vi "Core.vi"(0 "Image In":T12(plugin-control), 1 "CalibratedImage In":T12(plugin-control), 2 "Measurement JSON Data":T9 {"Ref ROI Cluster"."Edge Options ROI Ref"."Edge Polarity" items=["All Edges", "Rising Edges", "Falling Edges"]; "Ref ROI Cluster"."Edge Options ROI Ref"."Minimum Edge Strength" format="%.2f"; "Ref ROI Cluster"."Edge Options ROI Ref"."Width" step=2; "Ref ROI Cluster"."Edge Options ROI Ref"."Kernel Size" step=2; "Ref ROI Cluster"."Line Options ROI Ref"."Min. Points (%)" min=0.0 max=100.0; "Ref ROI Cluster"."Line Options ROI Ref"."Min. SNR (db)" min=0.0; "Ref ROI Cluster"."Line Options ROI Ref"."Max. Score" min=0.0 max=1024.0; "Ref ROI Cluster"."Line Options ROI Ref"."Min. Score" min=0.0 max=1024.0 step=1.0; "Measurement ROI 1 Cluster"."Meas ROI 1"."Contours"."Type" items=["No Selection", "Point", "Line", "Rectangle", "Oval", "Polygon", "Freehand Region", "Annulus", "Unused2", "Unused3", "Broken Line", "Freehand Line", "Rotated Rectangle"]; "Measurement ROI 1 Cluster"."Edge Options ROI 1"."Edge Polarity" items=["All Edges", "Rising Edges", "Falling Edges"]; "Measurement ROI 1 Cluster"."Edge Options ROI 1"."Minimum Edge Strength" format="%.2f"; "Measurement ROI 1 Cluster"."Edge Options ROI 1"."Width" step=2; "Measurement ROI 1 Cluster"."Edge Options ROI 1"."Kernel Size" step=2; "Measurement ROI 1 Cluster"."Line Options ROI 1"."Min. Points (%)" min=0.0 max=100.0; "Measurement ROI 1 Cluster"."Line Options ROI 1"."Min. SNR (db)" min=0.0; "Measurement ROI 1 Cluster"."Line Options ROI 1"."Max. Score" min=0.0 max=1024.0; "Measurement ROI 1 Cluster"."Line Options ROI 1"."Min. Score" min=0.0 max=1024.0 step=1.0; "Measurement ROI 1 Cluster"."Circle Options ROI 1"."Edge Options"."Edge Polarity" items=["All Edges", "Rising Edges", "Falling Edges"]; "Measurement ROI 1 Cluster"."Circle Options ROI 1"."Edge Options"."Minimum Edge Strength" format="%.2f"; "Measurement ROI 1 Cluster"."Circle Options ROI 1"."Edge Options"."Width" step=2; "Measurement ROI 1 Cluster"."Circle Options ROI 1"."Edge Options"."Kernel Size" step=2; "Measurement ROI 2 Cluster"."Meas ROI 2"."Contours"."Type" items=["No Selection", "Point", "Line", "Rectangle", "Oval", "Polygon", "Freehand Region", "Annulus", "Unused2", "Unused3", "Broken Line", "Freehand Line", "Rotated Rectangle"]; "Measurement ROI 2 Cluster"."Edge Options ROI 2"."Edge Polarity" items=["All Edges", "Rising Edges", "Falling Edges"]; "Measurement ROI 2 Cluster"."Edge Options ROI 2"."Minimum Edge Strength" format="%.2f"; "Measurement ROI 2 Cluster"."Edge Options ROI 2"."Width" step=2; "Measurement ROI 2 Cluster"."Edge Options ROI 2"."Kernel Size" step=2; "Measurement ROI 2 Cluster"."Line Options ROI 2"."Min. Points (%)" min=0.0 max=100.0; "Measurement ROI 2 Cluster"."Line Options ROI 2"."Min. SNR (db)" min=0.0; "Measurement ROI 2 Cluster"."Line Options ROI 2"."Max. Score" min=0.0 max=1024.0; "Measurement ROI 2 Cluster"."Line Options ROI 2"."Min. Score" min=0.0 max=1024.0 step=1.0; "Measurement ROI 2 Cluster"."Circle Options ROI 2"."Edge Options"."Edge Polarity" items=["All Edges", "Rising Edges", "Falling Edges"]; "Measurement ROI 2 Cluster"."Circle Options ROI 2"."Edge Options"."Minimum Edge Strength" format="%.2f"; "Measurement ROI 2 Cluster"."Circle Options ROI 2"."Edge Options"."Width" step=2; "Measurement ROI 2 Cluster"."Circle Options ROI 2"."Edge Options"."Kernel Size" step=2}, 3 "Transformed ROI cluster":T3 {"ROI Ref [ After Transformation]"."Contours"."Type" items=["No Selection", "Point", "Line", "Rectangle", "Oval", "Polygon", "Freehand Region", "Annulus", "Unused2", "Unused3", "Broken Line", "Freehand Line", "Rotated Rectangle"]; "Measurement ROI 1 [After Transformation]"."Contours"."Type" items=["No Selection", "Point", "Line", "Rectangle", "Oval", "Polygon", "Freehand Region", "Annulus", "Unused2", "Unused3", "Broken Line", "Freehand Line", "Rotated Rectangle"]; "Measurement ROI 2 [After Transformation]"."Contours"."Type" items=["No Selection", "Point", "Line", "Rectangle", "Oval", "Polygon", "Freehand Region", "Annulus", "Unused2", "Unused3", "Broken Line", "Freehand Line", "Rotated Rectangle"]}, 4 "Coordinate Other Cluster":T4, 5 "error in (no error)":errorcluster, 6 "coordinate system":T1) -> (13 "Overlay Arrow Lines":T11, 14 "Numeric":sgl, 19 "error out":errorcluster)   [LabVIEW 2019, in "Algorithm.lvclass"]
uses:
  FrameworkOverrides/Algorithm.lvclass
  <vilib>/vision/Measure.llb/Edge Options.ctl
  <vilib>/vision/Measure.llb/Edge Polarity.ctl
  <vilib>/vision/Measure.llb/Straight Edge Options.ctl
  <vilib>/vision/Measure.llb/Straight Edge Process.ctl
  <vilib>/vision/NI_Vision_Development_Module.lvlib
panel:
  out "Circle Fit Options ROI 1":T10
  out "Real World Value":sgl
  out "Pixel Value":sgl
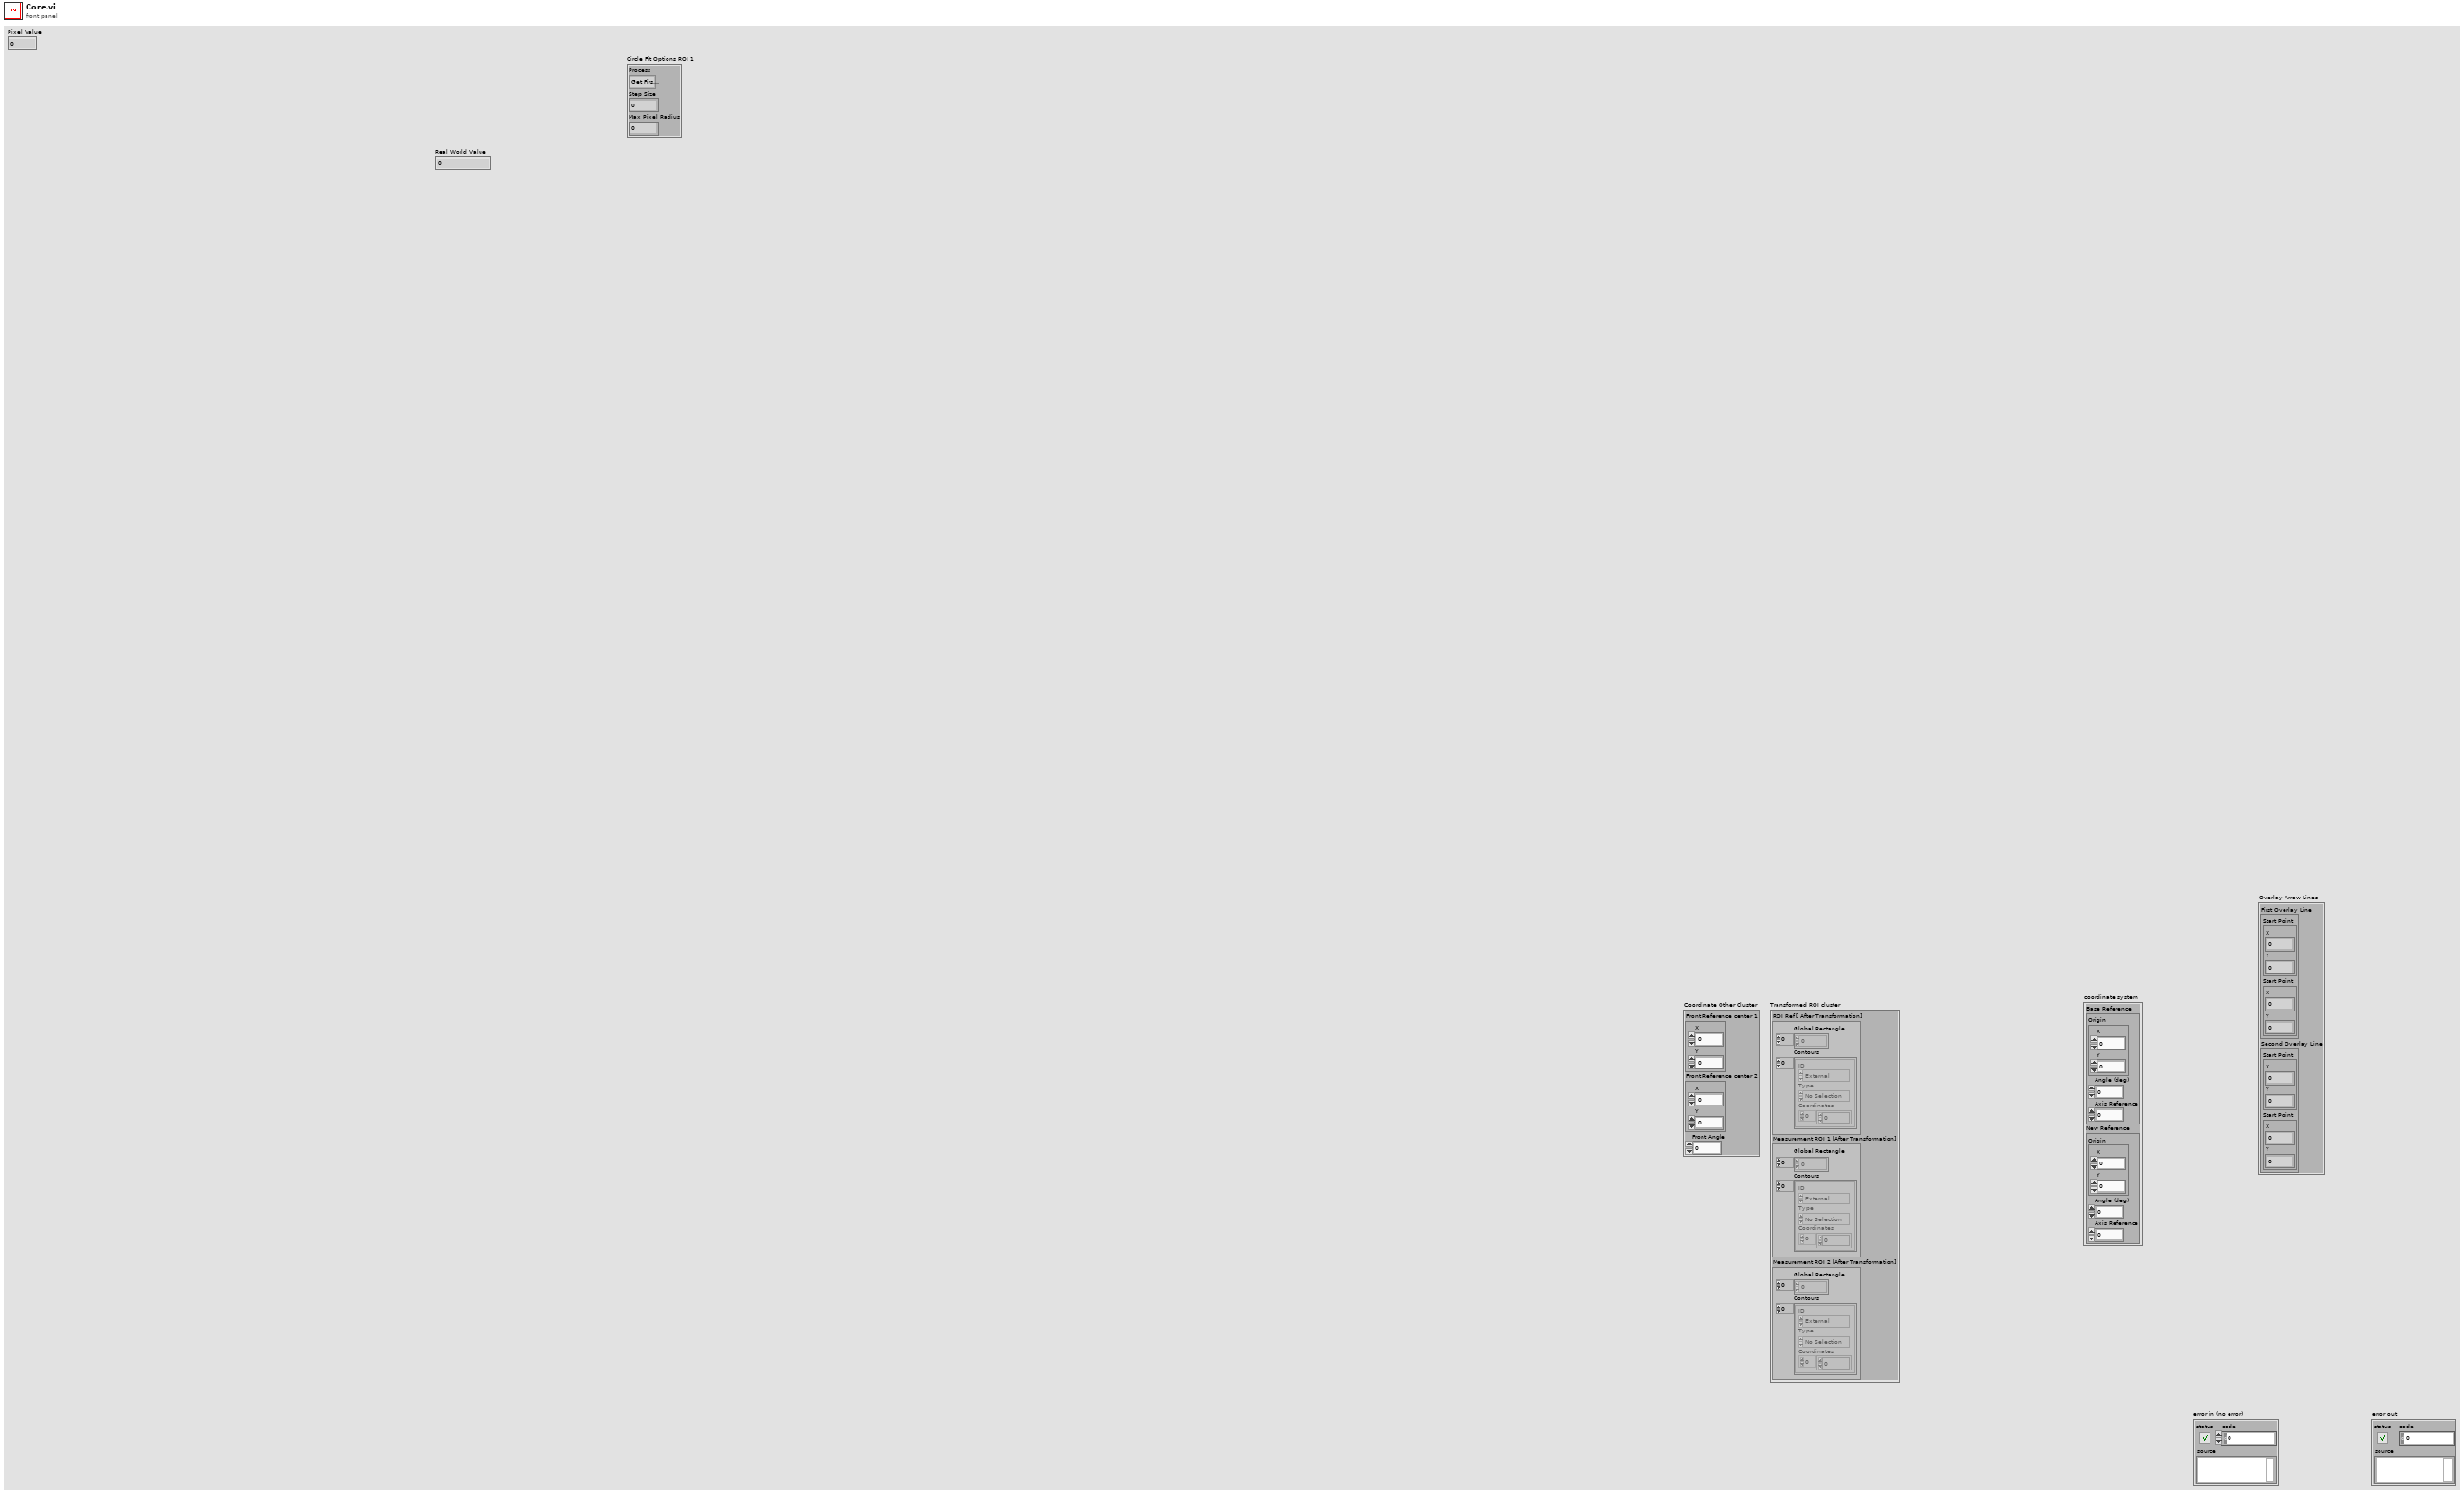
[diagram p1: front panel]
types:
  T1 = cluster{"Base Reference":cluster{"Origin":cluster{"X":sgl, "Y":sgl}, "Angle (deg)":sgl, "Axis Reference":u32}, "New Reference":cluster{"Origin":cluster{"X":sgl, "Y":sgl}, "Angle (deg)":sgl, "Axis Reference":u32}}
  T2 = typedef "ROI Descriptor" = cluster{"Global Rectangle":i32[], "Contours":cluster{"ID":enum32{"External", "Internal"}, "Type":u32, "Coordinates":i32[]}[]}
  T3 = cluster{"ROI Ref [ After Transformation]":T2, "Measurement ROI 1 [After Transformation]":T2, "Measurement ROI 2 [After Transformation]":T2}
  T4 = cluster{"Front Reference center 1":cluster{"X":sgl, "Y":sgl}, "Front Reference center 2":cluster{"X":sgl, "Y":sgl}, "Front Angle":dbl}
  T5 = typedef "Edge Options.ctl" = cluster{"Edge Polarity":T6, "Kernel Size":u32, "Width":u32, "Minimum Edge Strength":sgl, "Interpolation Type":enum32{"Zero Order", "Bilinear", "Quadratic", "Cubic", "Bilinear Fixed"}, "Data Processing Method":enum32{"Average", "Median"}}
  T6 = typedef "Edge Polarity.ctl" = u32
  T7 = typedef "Straight Edge Options.ctl" = cluster{"Number of Lines":i32, "Type":T8, "Min. Score":dbl, "Max. Score":dbl, "Orientation":dbl, "Angle Range":dbl, "Angle Tolerance":dbl, "Step Size":u32, "Min. SNR (db)":dbl, "Min. Points (%)":dbl, "Hough Iterations":i32}
  T8 = typedef "Straight Edge Process.ctl" = enum32{"First Edge Rake", "Best Edge Rake", "Hough Edge Rake", "First Edge Projection", "Best Edge Projection"}
  T9 = cluster{"RackID":i32, "ImageID":i32, "CameraID":i32, "MeasurementID":i32, "Measurement Name":string, "Algo Name":string, "Algo Type":string, "Ref ROI Cluster":cluster{"ROI Ref":cluster{"Global Rectangle":i32[], "Contours":cluster{"ID":enum32{"External", "Internal"}, "Type":u32, "Coordinates":i32[]}[]}, "Edge Options ROI Ref":T5, "Line Options ROI Ref":T7, "Search Direction ROI Ref":u32, "RefROIEnable":bool}, "Measurement ROI 1 Cluster":cluster{"Meas ROI 1":T2, "Edge Options ROI 1":T5, "Line Options ROI 1":T7, "Scan/Search Direction ROI 1":u16, "Step Size ROI 1":u32, "Process ROI 1":enum16{"Get First Edge", "Get First + Last Edge", "Get All Edges", "Get Best Edge"}, "Circle Options ROI 1":cluster{"Search  Direction":u32, "Edge Options":T5, "Show Search Area":bool, "Show Search Lines":bool, "Show Edges Found":bool, "Show Result":bool, "Search Area Color":u32, "Search Lines Color":u32, "Edge Locations Color":u32, "Result Color":u32, "Overlay Group Name":string}, "Circle Fit Options ROI 1":cluster{"Process":enum16{"Get First Edge", "Get First + Last Edge", "Get All Edges", "Get Best Edge"}, "Step Size":dbl, "Max Pixel Radius":i32}}, "Measurement ROI 2 Cluster":cluster{"Meas ROI 2":T2, "Edge Options ROI 2":T5, "Line Options ROI 2":T7, "Scan/Search Direction ROI 2":u32, "Step Size ROI 2":u32, "Process ROI 2":enum16{"Get First Edge", "Get First + Last Edge", "Get All Edges", "Get Best Edge"}, "Circle Options ROI 2":cluster{"Search  Direction":u32, "Edge Options":T5, "Show Search Area":bool, "Show Search Lines":bool, "Show Edges Found":bool, "Show Result":bool, "Search Area Color":u32, "Search Lines Color":u32, "Edge Locations Color":u32, "Result Color":u32, "Overlay Group Name":string}, "Circle Fit Options ROI 2":cluster{"Process":enum16{"Get First Edge", "Get First + Last Edge", "Get All Edges", "Get Best Edge"}, "Step Size":dbl, "Max Pixel Radius":i32}}, "OverlayOptions":cluster{"OverlayEnable":bool, "OverlayText":string, "OverlayCoords":i32[], "OverlayAngle":i32, "OverlayTextSize":i32, "OverlayTextColor":string, "OverlayROI":bool, "OverlayRakeLine":bool, "OverlayPoints":bool}, "MathExpression":cluster{"Algorithm":string, "MathExpression":string, "ResultVariable":string}, "MathCorrectionParameters":cluster{"Radius":dbl, "CurlGap":dbl, "Thickness":dbl, "MeasurementIndices":i32[], "MathAlgoName":string, "MathAlgoFormula":string, "CorrectionForAngle":i32[], "NumericAray":i32[], "StringArray":string[]}, "ResultVariableCluster":cluster{"RVName":string, "RVSequence":string, "RVIndex":i32, "RVID":i32, "RVValue":dbl}, "CalibrationCoefficients":cluster{"A1":dbl, "A2":dbl, "A3":dbl}, cluster{"UserCalibCoefficients":cluster{"UserCorrectionLinearityCoeff":dbl, "UserCorrectionBiasCoeff":dbl}}, "SpecValues":cluster{"LCL":dbl, "UCL":dbl, "LSL":dbl, "USL":dbl, "NominalValue":dbl}}
  T10 = cluster{"Process":enum16{"Get First Edge", "Get First + Last Edge", "Get All Edges", "Get Best Edge"}, "Step Size":dbl, "Max Pixel Radius":i32}
  T11 = cluster{"First Overlay Line ":cluster{"Start Point":cluster{"X":sgl, "Y":sgl}, "Start Point":cluster{"X":sgl, "Y":sgl}}, "Second Overlay Line ":cluster{"Start Point":cluster{"X":sgl, "Y":sgl}, "Start Point":cluster{"X":sgl, "Y":sgl}}}
  T12 = typedef "IMAQ Image.ctl" = refnum<image>
  T13 = cluster{"Contrast":i32, "Filter width":i32, "Steepness":i32, "Subsampling Ratio":u32, "Show Search Area":bool, "Show Search Lines":bool, "Show Edges Found":bool, "Show Result":bool}
  T14 = cluster{"AvgMinMax":enum16{"Average", "Max", "Min", "Max2"}, "Center X &Y":cluster{"Center X":dbl, "Center Y":dbl}, "Reference ROI Before Transformation":T2, "Measurement ROI-1 Before transformation":T2, "Ref Line Edge Options":T5, "Ref Line Search Direction":u32, "Ref Line Options":T7, "Meas ROI-1 Edge Options":T5, "Meas ROI-1 Step Size":u32, "Meas ROI-1 Scan Direction":u16, "Meas ROI-1 Process":enum16{"Get First Edge", "Get First + Last Edge", "Get All Edges", "Get Best Edge"}, "OverlayOptions":cluster{"OverlayEnable":bool, "OverlayText":string, "OverlayCoords":i32[], "OverlayAngle":i32, "OverlayTextSize":i32, "OverlayTextColor":string, "OverlayROI":bool, "OverlayRakeLine":bool, "OverlayPoints":bool}}
  T15 = cluster{"ROI 2 Descriptor":T2, " ROI 2 Step Size":u32, "ROI 2 Scan Direction":u16, "ROI 2 Process":enum16{"Get First Edge", "Get First + Last Edge", "Get All Edges", "Get Best Edge"}, "ROI 2 Edge Options":T5, "ROI 2 Overlay":bool, "ROI 2 Rake Line Overlay":bool, "ROI 2 Edge/Point Overlay":bool}
  T16 = cluster{"ROI 1 Descriptor":cluster{"Global Rectangle":i32[], "Contours":cluster{"ID":enum32{"External", "Internal"}, "Type":u32, "Coordinates":i32[]}[]}, "ROI 1 Line Options":T7, "ROI 1 Edge Options":T5, "ROI 1 Search Direction":u32, "ROI 1 Overlay":bool, "ROI 1 Rake Line Overlay":bool, "ROI 1 Edge/Point Overlay":bool}
  T17 = cluster{"ROI 2 After Transformation":cluster{"Global Rectangle":i32[], "Contours":cluster{"ID":enum32{"External", "Internal"}, "Type":u32, "Coordinates":i32[]}[]}, "ROI 2 Edge Options":T5, "ROI 2 Scan Direction":u16, "ROI 2 Step Size":u32, "ROI 2 Process":enum16{"Get First Edge", "Get First + Last Edge", "Get All Edges", "Get Best Edge"}, "ROI 2 Overlay":bool, "ROI 2 Rake Line Overlay":bool, "ROI 2 Edge/Point Overlay":bool}
  T18 = cluster{"ROI 1 After Transformation":cluster{"Global Rectangle":i32[], "Contours":cluster{"ID":enum32{"External", "Internal"}, "Type":u32, "Coordinates":i32[]}[]}, "ROI 1 Edge Options":T5, "ROI 1 Scan Direction":u16, "ROI 1 Step Size":u32, "ROI 1 Process":enum16{"Get First Edge", "Get First + Last Edge", "Get All Edges", "Get Best Edge"}, "ROI 1 Overlay":bool, "ROI 1 Rake Line Overlay":bool, "ROI 1 Edge/Point Overlay":bool}
  T19 = cluster{"Ref ROI After Transformation":cluster{"Global Rectangle":i32[], "Contours":cluster{"ID":enum32{"External", "Internal"}, "Type":u32, "Coordinates":i32[]}[]}, "Ref ROI Edge Options":T5, "Ref ROI Line Options":T7, "Ref ROI Search Direction":u32, "Ref ROI Overlay":bool}
  T20 = cluster{"Point 2":cluster{"X":sgl, "Y":sgl}, "Start Point":cluster{"X":sgl, "Y":sgl}}
  T21 = cluster{"Start Point":cluster{"X":sgl, "Y":sgl}, "Point 1":cluster{"X":sgl, "Y":sgl}}
  T22 = cluster{"First Overlay Line ":cluster{"Start Point":cluster{"X":sgl, "Y":sgl}, "Point 1":cluster{"X":sgl, "Y":sgl}}, "Second Overlay Line ":cluster{"Point 2":cluster{"X":sgl, "Y":sgl}, "Start Point":cluster{"X":sgl, "Y":sgl}}}
  T23 = cluster{"Search Direction":u32, "Edge Options":T5, "Show Search Area":bool, "Show Search Lines":bool, "Show Edges Found":bool, "Show Result":bool, "Search Area Color":u32, "Search Lines Color":u32, "Edge Locations Color":u32, "Result Color":u32, "Overlay Group Name":string}
  T24 = enum16{"Get First Edge", "Get First + Last Edge", "Get All Edges", "Get Best Edge"}
  T25 = cluster{"First Overlay Line ":cluster{"Start Point":cluster{"X":sgl, "Y":sgl}, "Intersection Point":cluster{"X":sgl, "Y":sgl}}, "Second Overlay Line ":cluster{"Intersection Point":cluster{"X":sgl, "Y":sgl}, "Start Point":cluster{"X":sgl, "Y":sgl}}}
  T26 = cluster{"First Overlay Line ":cluster{"Point 1":cluster{"X":sgl, "Y":sgl}, "Point 1":cluster{"X":sgl, "Y":sgl}}, "Second Overlay Line ":cluster{"Point 2":cluster{"X":sgl, "Y":sgl}, "Point 1":cluster{"X":sgl, "Y":sgl}}}
  T27 = cluster{"ROI 1 Before Transformation":cluster{"Global Rectangle":i32[], "Contours":cluster{"ID":enum32{"External", "Internal"}, "Type":u32, "Coordinates":i32[]}[]}, "ROI 1 Scan Direction":u16, "ROI 1 Edge Options":T5, "ROI 1Step Size":u32, "ROI 1 Process":enum16{"Get First Edge", "Get First + Last Edge", "Get All Edges", "Get Best Edge"}, "ROI 1 Overlay":bool, "ROI 1 Rake Line Overlay":bool, "ROI 1 Edge/Point Overlay":bool}
  T28 = cluster{"Ref Line ROI Before Transformation":cluster{"Global Rectangle":i32[], "Contours":cluster{"ID":enum32{"External", "Internal"}, "Type":u32, "Coordinates":i32[]}[]}, "Ref ROI Search Direction":u32, "Ref ROI Edge Options":T5, "Ref ROI Line Options":T7, "Ref ROI Overlay":bool, "Ref Rake Line Overlay 2":bool, "Ref Edge/Point Overlay":bool}
  T29 = cluster{"Overlay ROI":bool, "Overlay Edge/ Points":bool, "Overlay Rake Lines":bool}
  T30 = cluster{"1629 side E Ref ROI before transformation":T2, "Ref Search Direction":u32, "Ref Edge Options":T5, "Ref Line Options":T7, "Meas ROI-1 Descriptor before transformation":T2, "Meas-1 Step Size":u32, "Meas-1 Scan Direction":u16, "Meas-1 Edge Options":T5, "Meas ROI-2 Descriptor Before Transformation":T2, "Meas-2 Scan Direction":u32, "Meas-2 Edge Options":T5, "Meas-2 Line Options":T7, "Ellipse Center":cluster{"X":sgl, "Y":sgl}}
  T31 = cluster{"OverlayEnable":bool, "OverlayText":string, "OverlayCoords":i32[], "OverlayAngle":i32, "OverlayTextSize":i32, "OverlayTextColor":string, "OverlayROI":bool, "OverlayRakeLine":bool, "OverlayPoints":bool}
  T32 = typedef "Edge New.ctl" = cluster{"Location (Pixel)":cluster{"X":sgl, "Y":sgl}, "Location (Real-World)":cluster{"X":sgl, "Y":sgl}, "Distance (Pixel)":dbl, "Distance (Real-World)":dbl, "Strength":dbl, "Noise":dbl, "Rising?":bool}
  T33 = typedef "Search Line.ctl" = cluster{"Start Point":cluster{"X":sgl, "Y":sgl}, "End Point":cluster{"X":sgl, "Y":sgl}, "Edge Info":T32[], "Edge Map":dbl[], "Calibration Valid":bool}
  T34 = cluster{"Start Point":cluster{"X":sgl, "Y":sgl}, "Location (Pixel)":cluster{"X":sgl, "Y":sgl}, "Location (Pixel)":cluster{"X":sgl, "Y":sgl}, "End Point":cluster{"X":sgl, "Y":sgl}}
  T35 = typedef "IMAQ Rectangle" = cluster{"Left":i32, "Top":i32, "Right":i32, "Bottom":i32, "Rotation":dbl}
  T36 = cluster{"element":cluster{"X":sgl, "Y":sgl}, cluster{"X":sgl, "Y":sgl}, cluster{"X":sgl, "Y":sgl}, "element":cluster{"X":sgl, "Y":sgl}}
  T37 = cluster{"element":cluster{"X":sgl, "Y":sgl}, "element":cluster{"X":sgl, "Y":sgl}}
  T38 = cluster{"Origin":cluster{"X":sgl, "Y":sgl}, "Angle (deg)":sgl, "Axis Reference":u32}
  T39 = cluster{"Global Rectangle":i32[], "Contours":cluster{"ID":enum32{"External", "Internal"}, "Type":u32, "Coordinates":i32[]}[]}
  T40 = cluster{"L":dbl, "Line Coordinates":cluster{"Point1":cluster{"X":sgl, "Y":sgl}, "Point2":cluster{"X":sgl, "Y":sgl}}}
  T41 = cluster{"L Meas":sgl, "output cluster":cluster{"Point 2":cluster{"X":sgl, "Y":sgl}, "Point 2":cluster{"X":sgl, "Y":sgl}}}
  T42 = cluster{cluster{cluster{sgl, "Y":sgl}, "Point 2":cluster{"X":sgl, "Y":sgl}}, cluster{"Point 2":cluster{"X":sgl, "Y":sgl}, cluster{sgl, "Y":sgl}}}
  T43 = cluster{"Point1 (Pixels)":cluster{"X":sgl, "Y":sgl}, "Point2 (Pixels)":cluster{"X":sgl, "Y":sgl}, "Point1 (Real-World)":cluster{"X":sgl, "Y":sgl}, "Point2 (Real-World)":cluster{"X":sgl, "Y":sgl}, "Angle (Pixel)":dbl, "Angle (Real-World)":dbl, "Score":dbl, "Straightness":dbl, "Average SNR (db)":dbl, "Calibration Valid":bool}[]
  T44 = cluster{"Point1 (Pixels)":cluster{"X":sgl, "Y":sgl}, "Point2 (Pixels)":cluster{"X":sgl, "Y":sgl}, "Point1 (Real-World)":cluster{"X":sgl, "Y":sgl}, "Point2 (Real-World)":cluster{"X":sgl, "Y":sgl}, "Angle (Pixel)":dbl, "Angle (Real-World)":dbl, "Score":dbl, "Straightness":dbl, "Average SNR (db)":dbl, "Calibration Valid":bool}
  T45 = cluster{"Point1 (Pixels)":cluster{"X":sgl, "Y":sgl}, "Point2 (Pixels)":cluster{"X":sgl, "Y":sgl}}
  T46 = cluster{"Point 1":cluster{"X":sgl, "Y":sgl}, "Point 2":cluster{"X":sgl, "Y":sgl}}
  T47 = cluster{"Search  Direction":u32, "Edge Options":T5, "Show Search Area":bool, "Show Search Lines":bool, "Show Edges Found":bool, "Show Result":bool, "Search Area Color":u32, "Search Lines Color":u32, "Edge Locations Color":u32, "Result Color":u32, "Overlay Group Name":string}
  T48 = typedef "IMAQ Circle" = cluster{"Center X":i32, "Center Y":i32, "Inner Radius":i32, "Outer Radius":i32, "Start Angle":dbl, "End Angle":dbl}
  T49 = cluster{"Center (Pixels)":cluster{"X":sgl, "Y":sgl}, "Radius (Pixels)":dbl, "Center (Real-World)":cluster{"X":sgl, "Y":sgl}, "Radius (Real-World)":dbl, "Roundness (Real-World)":dbl, "Average Strength":dbl, "Average SNR (dB)":dbl}
  T50 = cluster{"Center (Pixels)":cluster{"X":sgl, "Y":sgl}, "Center (Pixels)":cluster{"X":sgl, "Y":sgl}}
  T51 = cluster{cluster{"Center (Pixels)":cluster{"X":sgl, "Y":sgl}, "Center (Pixels)":cluster{"X":sgl, "Y":sgl}}, cluster{"Center (Pixels)":cluster{"X":sgl, "Y":sgl}, "Center (Pixels)":cluster{"X":sgl, "Y":sgl}}}
  T52 = cluster{cluster{sgl, "Y":sgl}, cluster{"X":sgl, "Y":sgl}}
  T53 = cluster{cluster{"X":sgl, "Y":sgl}, cluster{sgl, "Y":sgl}}
  T54 = cluster{"Meas ROI 1":T2, "Edge Options ROI 1":T5, "Line Options ROI 1":T7, "Scan/Search Direction ROI 1":u16, "Step Size ROI 1":u32, "Process ROI 1":enum16{"Get First Edge", "Get First + Last Edge", "Get All Edges", "Get Best Edge"}, "Circle Options ROI 1":cluster{"Search  Direction":u32, "Edge Options":T5, "Show Search Area":bool, "Show Search Lines":bool, "Show Edges Found":bool, "Show Result":bool, "Search Area Color":u32, "Search Lines Color":u32, "Edge Locations Color":u32, "Result Color":u32, "Overlay Group Name":string}, "Circle Fit Options ROI 1":cluster{"Process":enum16{"Get First Edge", "Get First + Last Edge", "Get All Edges", "Get Best Edge"}, "Step Size":dbl, "Max Pixel Radius":i32}}
  T55 = cluster{"Meas ROI 2":T2, "Edge Options ROI 2":T5, "Line Options ROI 2":T7, "Scan/Search Direction ROI 2":u32, "Step Size ROI 2":u32, "Process ROI 2":enum16{"Get First Edge", "Get First + Last Edge", "Get All Edges", "Get Best Edge"}, "Circle Options ROI 2":cluster{"Search  Direction":u32, "Edge Options":T5, "Show Search Area":bool, "Show Search Lines":bool, "Show Edges Found":bool, "Show Result":bool, "Search Area Color":u32, "Search Lines Color":u32, "Edge Locations Color":u32, "Result Color":u32, "Overlay Group Name":string}, "Circle Fit Options ROI 2":cluster{"Process":enum16{"Get First Edge", "Get First + Last Edge", "Get All Edges", "Get Best Edge"}, "Step Size":dbl, "Max Pixel Radius":i32}}
  T56 = cluster{"ROI Ref":cluster{"Global Rectangle":i32[], "Contours":cluster{"ID":enum32{"External", "Internal"}, "Type":u32, "Coordinates":i32[]}[]}, "Edge Options ROI Ref":T5, "Line Options ROI Ref":T7, "Search Direction ROI Ref":u32, "RefROIEnable":bool}
  T57 = cluster{cluster{cluster{"X":sgl, sgl}, cluster{"X":sgl, "Y":sgl}}, cluster{"Location (Pixel)":cluster{"X":sgl, "Y":sgl}, cluster{"X":sgl, sgl}}}
  T58 = cluster{cluster{cluster{sgl, "Y":sgl}, "Intersection Point":cluster{"X":sgl, "Y":sgl}}, cluster{"Intersection Point":cluster{"X":sgl, "Y":sgl}, cluster{sgl, "Y":sgl}}}
  T59 = cluster{"E Side EMeasurement":sgl, "Points for Arrow Overlay":cluster{"X":sgl, "Y":sgl}[]}
  T60 = cluster{"End Point":cluster{"X":sgl, "Y":sgl}, "End Point":cluster{"X":sgl, "Y":sgl}}
  T61 = cluster{cluster{"End Point":cluster{"X":sgl, "Y":sgl}, "End Point":cluster{"X":sgl, "Y":sgl}}, cluster{"End Point":cluster{"X":sgl, "Y":sgl}, "End Point":cluster{"X":sgl, "Y":sgl}}}
  T62 = cluster{"Left":dbl, "Top":dbl, "Right":dbl, "Bottom":dbl, "Angle":dbl}
  T63 = cluster{cluster{"element":cluster{"X":sgl, "Y":sgl}, "element":cluster{"X":sgl, "Y":sgl}}, cluster{"element":cluster{"X":sgl, "Y":sgl}, "element":cluster{"X":sgl, "Y":sgl}}}
  T64 = cluster{cluster{cluster{"X":sgl, sgl}, "Point 1":cluster{"X":sgl, "Y":sgl}}, cluster{"Point 2":cluster{"X":sgl, "Y":sgl}, cluster{"X":sgl, sgl}}}
  T65 = cluster{"Points for Overlay":cluster{"X":sgl, "Y":sgl}[], "E1":sgl}
  T66 = cluster{"Point 1":cluster{"X":sgl, "Y":sgl}, "Point 1":cluster{"X":sgl, "Y":sgl}}
  T67 = cluster{cluster{"Point 1":cluster{"X":sgl, "Y":sgl}, "Point 1":cluster{"X":sgl, "Y":sgl}}, cluster{"Point 1":cluster{"X":sgl, "Y":sgl}, "Point 1":cluster{"X":sgl, "Y":sgl}}}
  T68 = cluster{cluster{cluster{sgl, "Y":sgl}, "Point 1":cluster{"X":sgl, "Y":sgl}}, cluster{"Point 2":cluster{"X":sgl, "Y":sgl}, cluster{sgl, "Y":sgl}}}
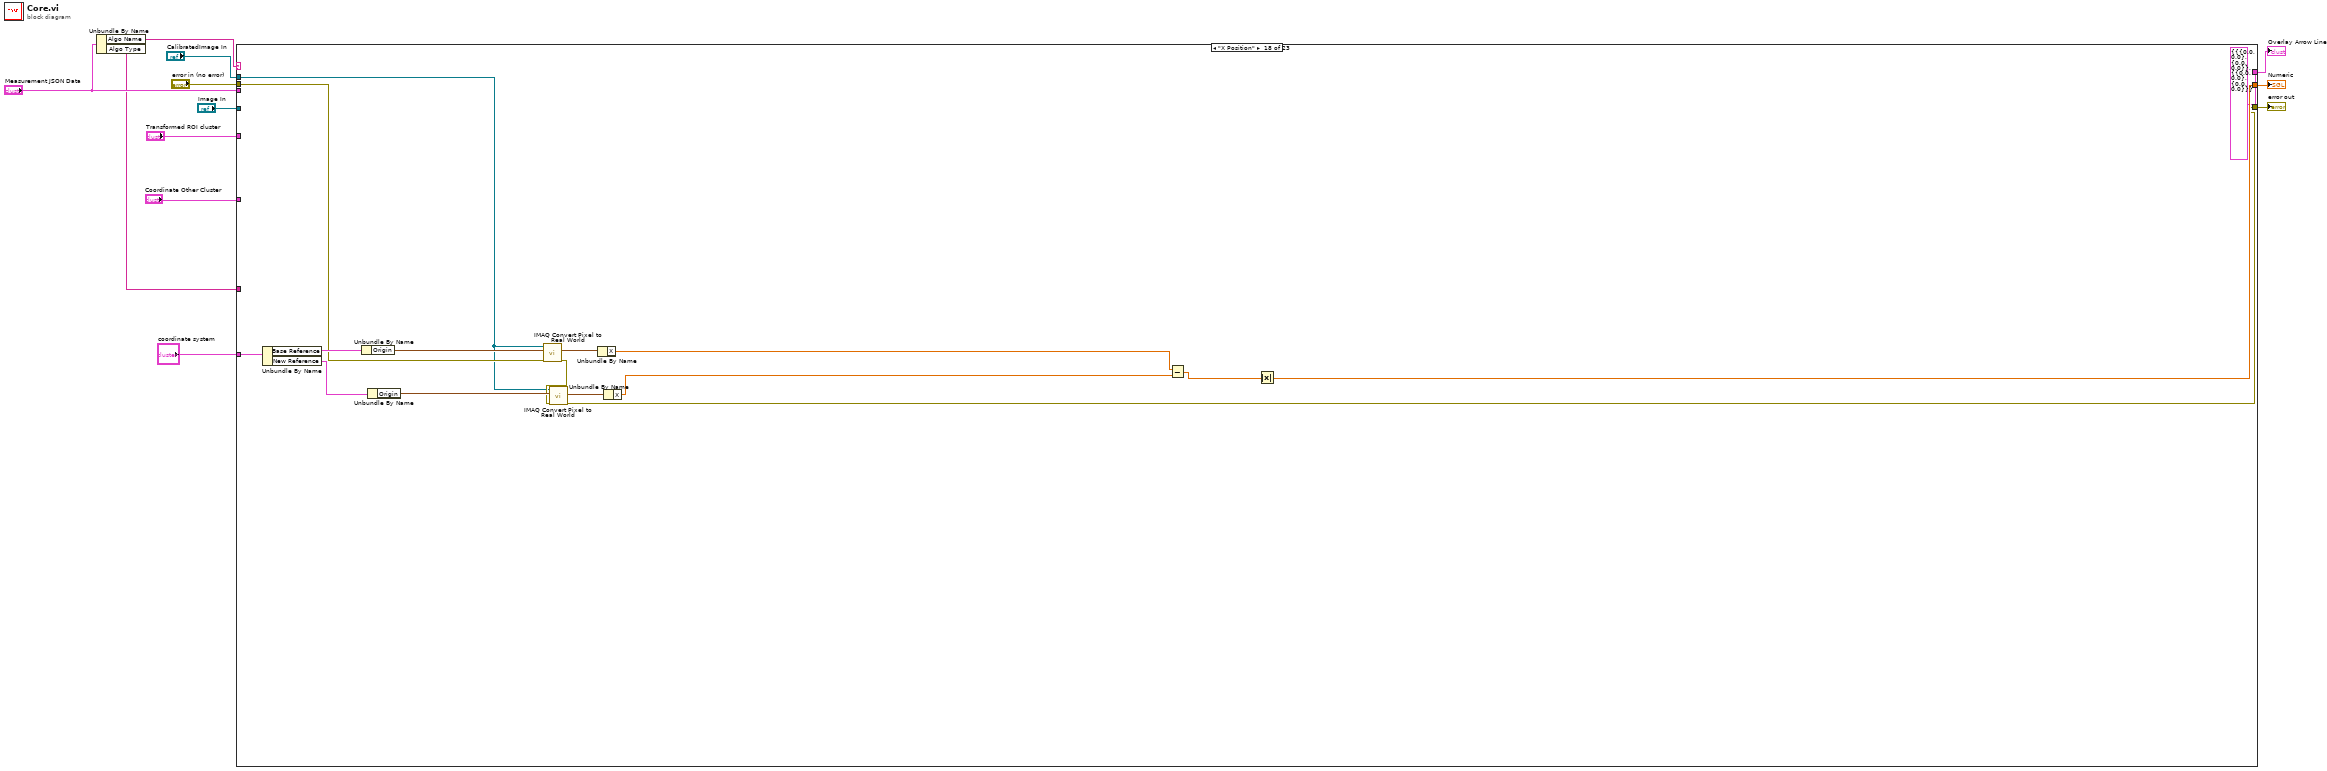
[diagram p0: block diagram]
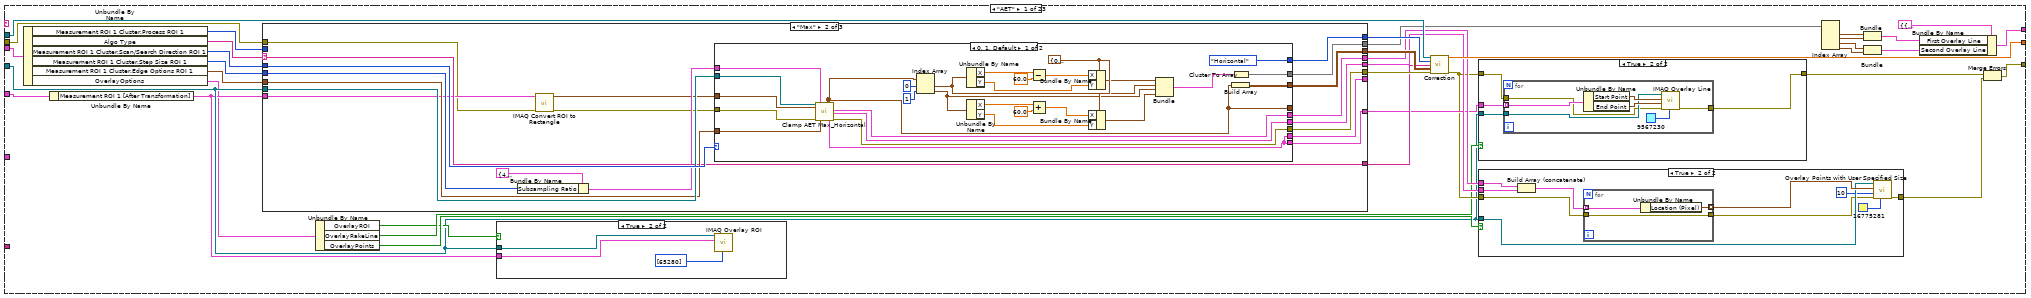
[diagram p2: hidden frame]
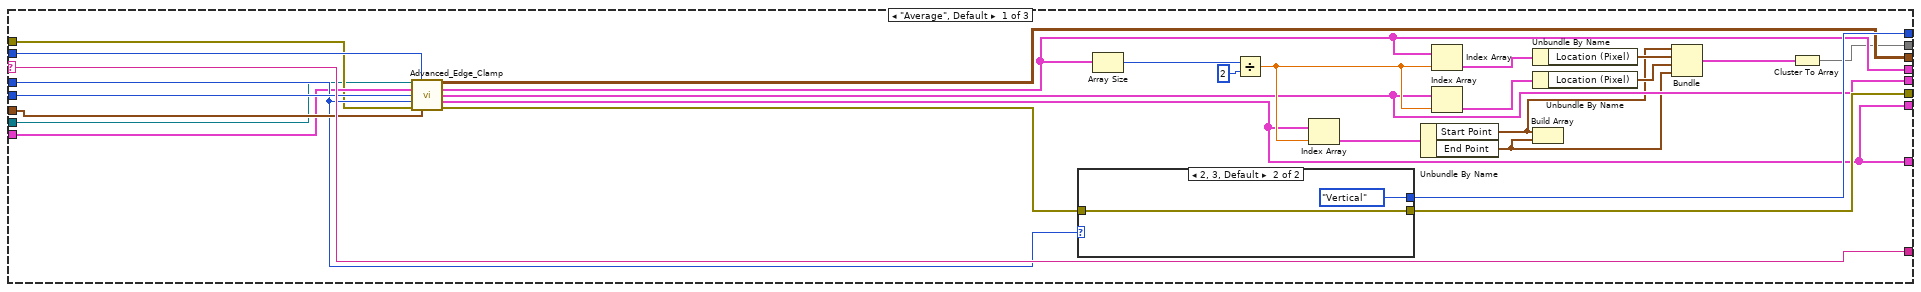
[diagram p6: hidden frame]
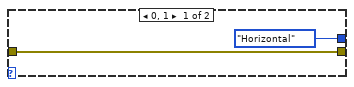
[diagram p7: hidden frame]
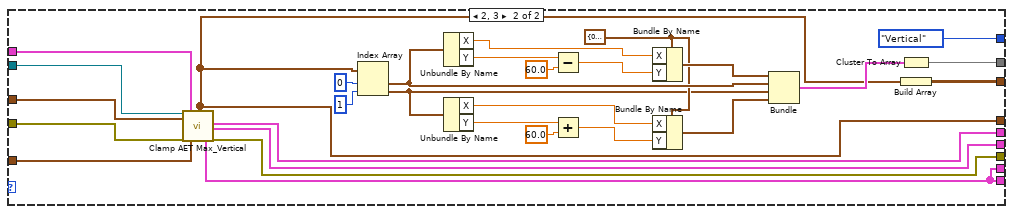
[diagram p8: hidden frame]
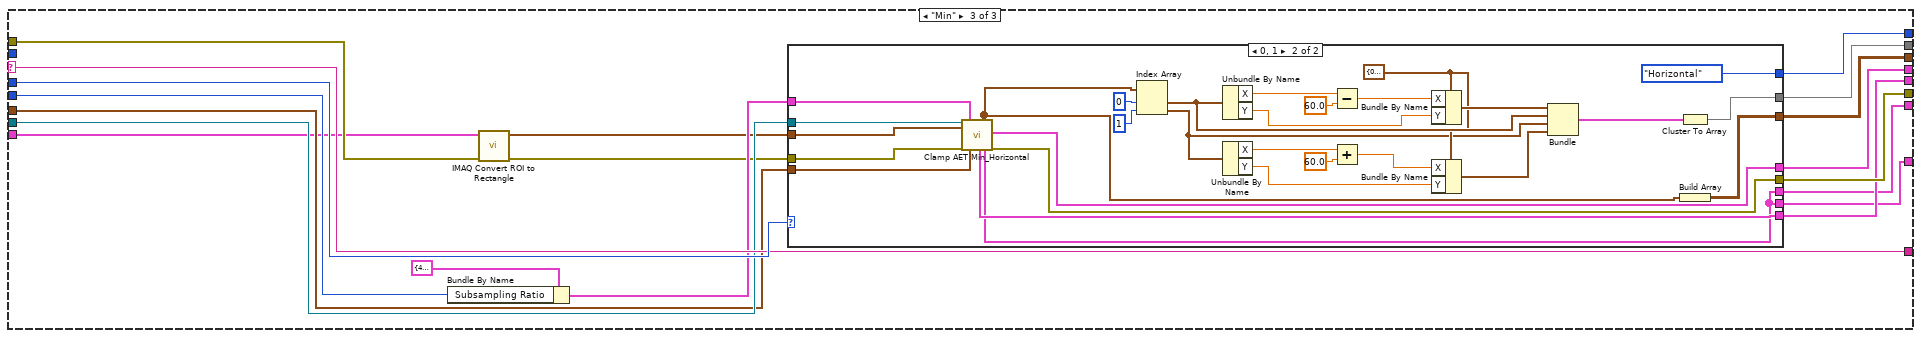
[diagram p9: hidden frame]
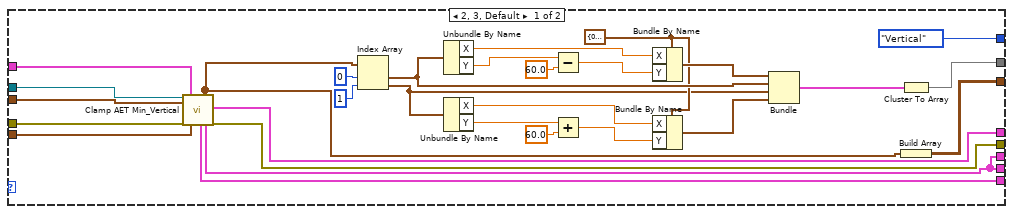
[diagram p10: hidden frame]
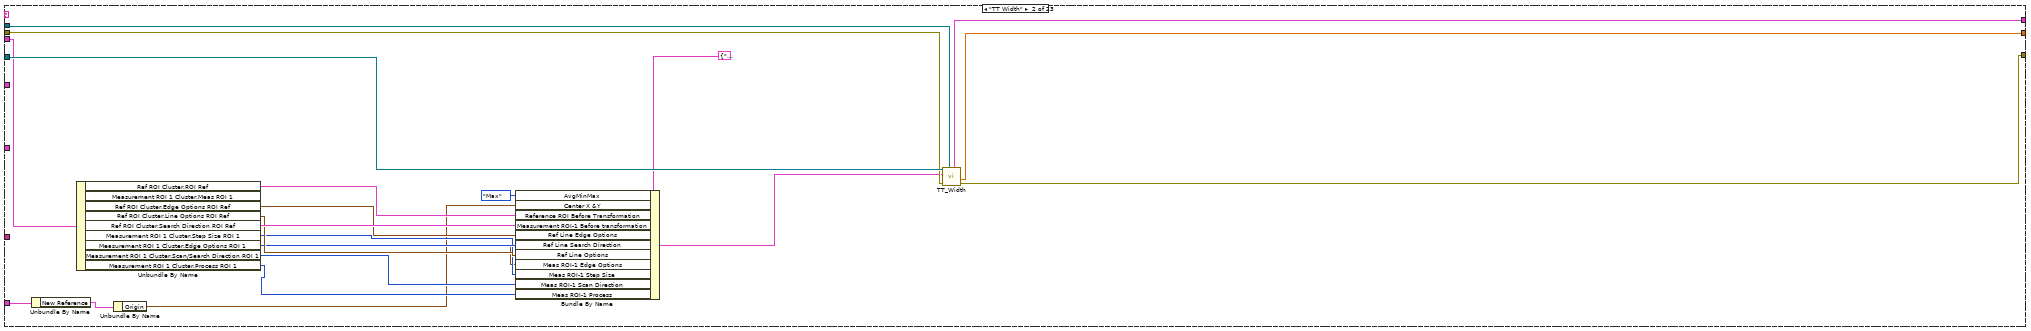
[diagram p11: hidden frame]
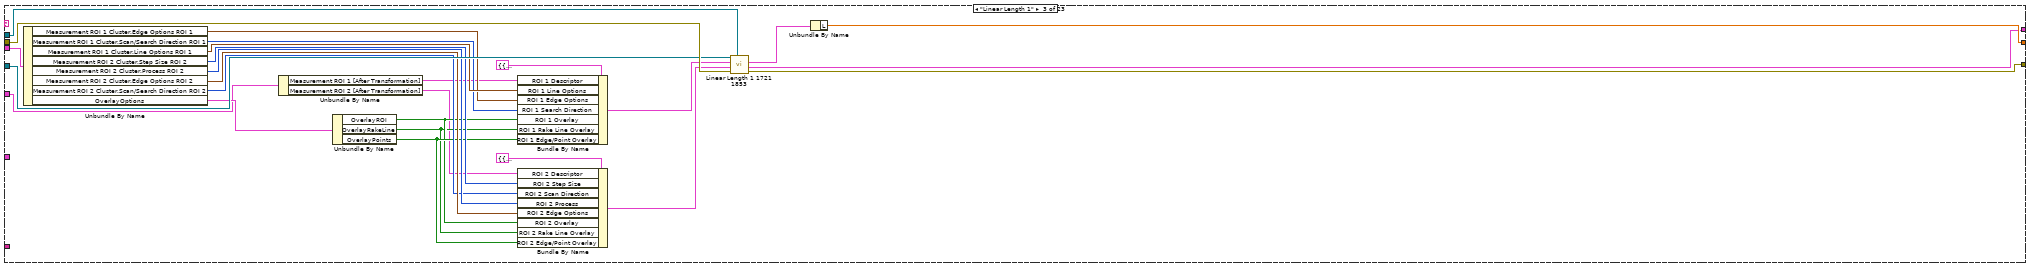
[diagram p12: hidden frame]
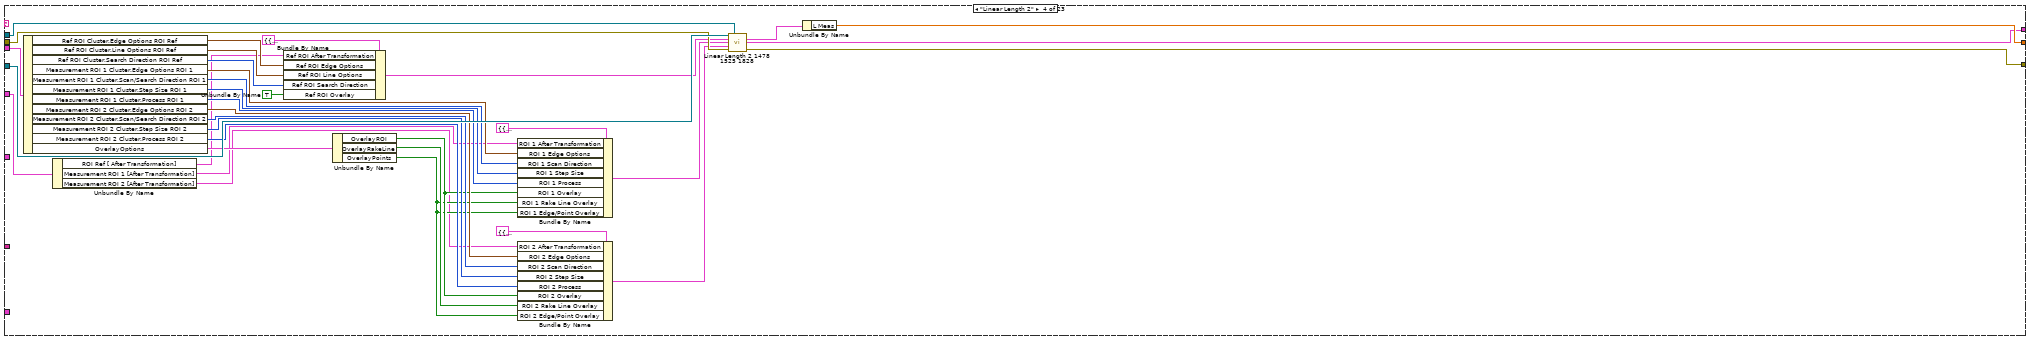
[diagram p13: hidden frame]
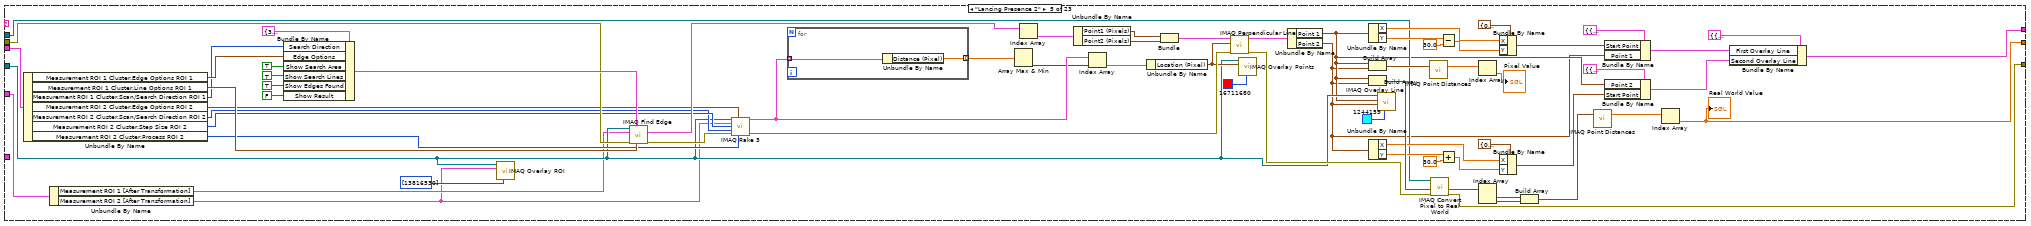
[diagram p14: hidden frame]
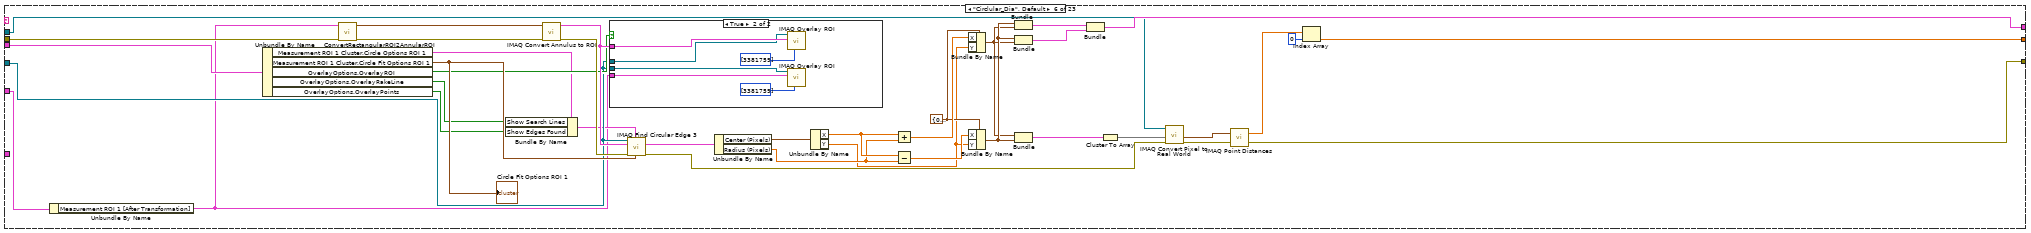
[diagram p15: hidden frame]
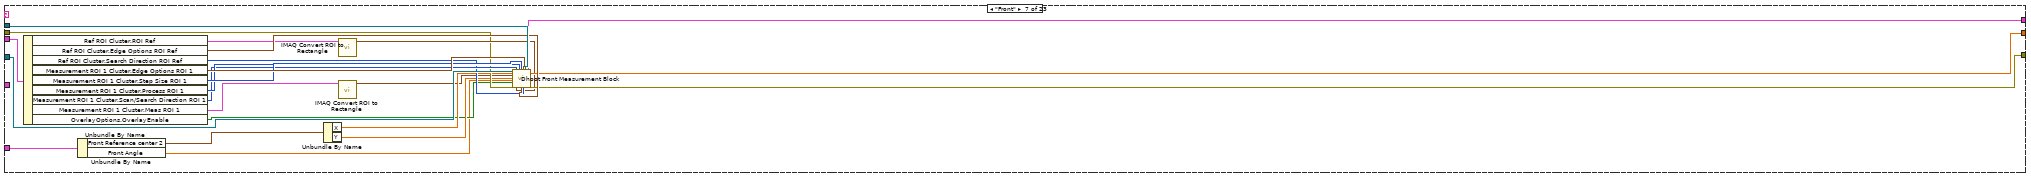
[diagram p17: hidden frame]
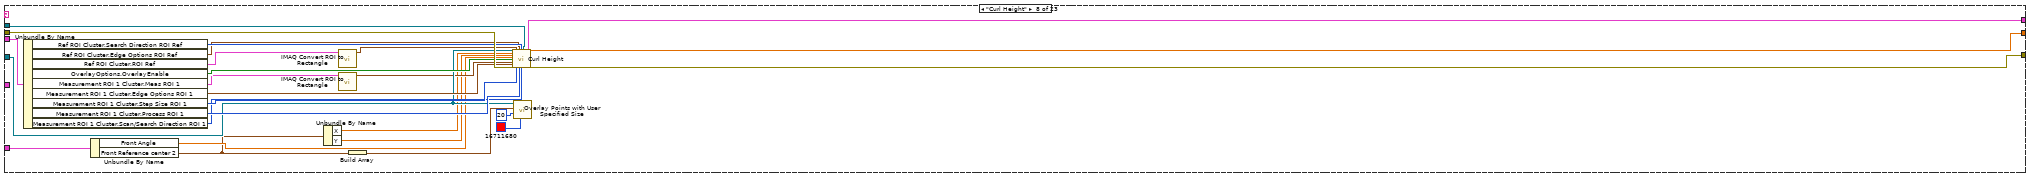
[diagram p18: hidden frame]
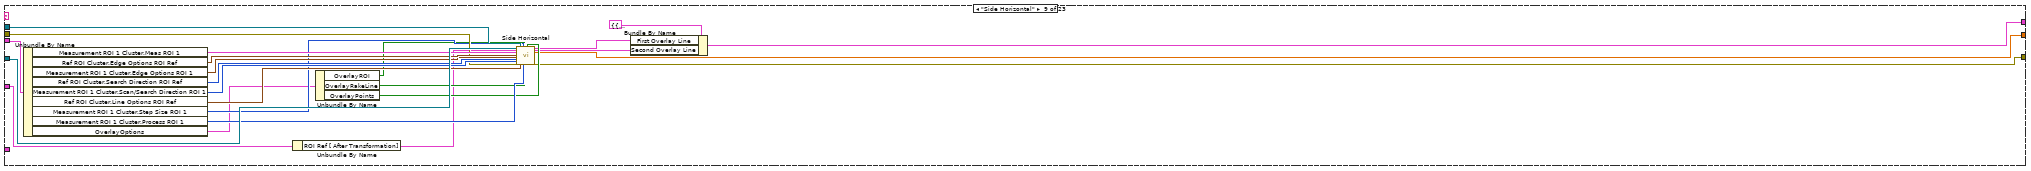
[diagram p19: hidden frame]
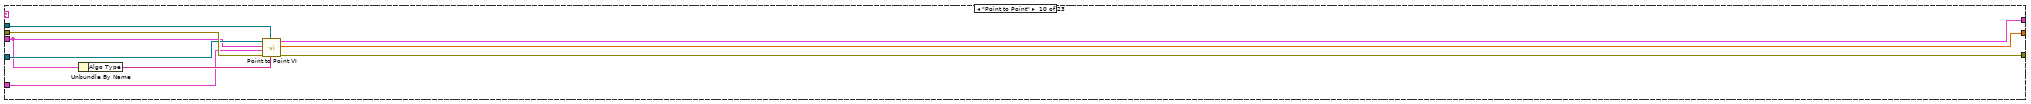
[diagram p20: hidden frame]
diagram:
  n1 = Unbundle By Name("Measurement JSON Data") -> ("Algo Name"=w6:string, "Algo Type"=w1:string)
  n2 = case shown="\"X Position\"" w6 {
    tunnel: "error in (no error)" -> [w40 w279 w306 w340 w380 w436 w466 w506 w523 w540 w549 w623 w633 w659 w669 w674 w689 w705 w751 w808 w818 w854 w889]
    tunnel: "CalibratedImage In" -> [w37 w283 w305 w341 w354 w423 w479 w505 w529 w538 w589 w626 w634 w655 _ w683 w685 w701 w750 w806 w823 w856 w887]
    tunnel: "Image In" -> [w26 w284 w304 w342 w353 w421 w480 w492 w530 w539 w561 w625 w635 w656 w670 w682 _ _ w749 w807 w822 w855 w888]
    tunnel: [w39 w281 w310 w344 w372 w435 w471 w497 w512 w532 w545 w621 w627 w652 w660 w673 w687 w703 w724 w785 w819 w839 w861] -> w9
    tunnel: "Measurement JSON Data" -> [w14 w275 w309 w343 w381 w432 w481 w507 w531 w537 _ w619 _ w649 w666 w679 _ _ w744 w791 w829 w852 w881]
    tunnel: [w30 w282 w308 w339 w355 w433 w472 w496 w511 w533 w580 w622 w629 w658 w661 w672 w686 w702 w725 w784 w820 w838 w863] -> w8
    tunnel: [w24 w280 w288 w315 w356 w425 w470 w495 w510 w534 w564 _ w628 w651 _ _ T25 {"First Overlay Line "={"Start Point"={"X"=0.0, "Y"=0.0}, "Intersection Point"={"X"=0.0, "Y"=0.0}}, "Second Overlay Line "={"Intersection Point"={"X"=0.0, "Y"=0.0}, "Start Point"={"X"=0.0, "Y"=0.0}}} ("overlay arrow lines") T26 {"First Overlay Line "={"Point 1"={"X"=0.0, "Y"=0.0}, "Point 1"={"X"=0.0, "Y"=0.0}}, "Second Overlay Line "={"Point 2"={"X"=0.0, "Y"=0.0}, "Point 1"={"X"=0.0, "Y"=0.0}}} ("Arrow Overlay lines") w716 w758 w821 w830 w862] -> w7
    tunnel: "Transformed ROI cluster" -> [w16 _ w287 w314 w347 w416 _ _ w509 w535 w541 w620 w632 w657 w668 w681 _ _ _ _ _ _ _]
    tunnel: "Coordinate Other Cluster" -> [_ _ _ _ _ _ w469 w486 _ _ _ _ _ _ _ _ _ _ _ _ _ _ _]
    tunnel: "coordinate system" -> [_ w265 _ _ _ _ _ _ _ _ _ _ _ _ _ _ w699 w715 w754 w805 w828 w858 w886]
    tunnel: w1 -> [_ _ _ _ _ _ _ _ _ _ _ _ _ _ _ _ _ _ w746 _ _ _ _]
    frame "AET" {
      n3 = Unbundle By Name(w14) -> ("Measurement ROI 1 Cluster.Process ROI 1"=w47:T24, "Algo Type"=w41:string, "Measurement ROI 1 Cluster.Scan/Search Direction ROI 1"=w42:u16, "Measurement ROI 1 Cluster.Step Size ROI 1"=w45:u32, "Measurement ROI 1 Cluster.Edge Options ROI 1"=w46:T5, "OverlayOptions"=w13:T31)
      n4 = Unbundle By Name(w16) -> ("Measurement ROI 1 [After Transformation]"=w15:T2)
      n5 = case shown="\"Max\"" w41 {
        selector: w41 -> [w104 w122 w203]
        tunnel: w42 -> [w97 w127 w204]
        tunnel: [w104 w122 w203] -> w38
        tunnel: [w103 w121 w194] -> w43
        tunnel: [w102 w123 w202] -> w44
        tunnel: w15 -> [w96 w117 w191]
        tunnel: w45 -> [w101 w119 w196]
        tunnel: w46 -> [w100 w124 w200]
        tunnel: w26 -> [w88 w126 w201]
        tunnel: w47 -> [w99 _ _]
        tunnel: [w98 w125 w199] -> w48
        tunnel: w40 -> [w95 w114 w193]
        tunnel: [w81 w113 w192] -> w23
        tunnel: [w86 w112 w189] -> w36
        tunnel: [w85 w111 w188] -> w35
        tunnel: [w78 w110 w187] -> w34
        tunnel: [w78 w109 w186] -> _
        frame "Average", Default {
          n6 = call "Advanced_Edge_Clamp.vi"("Image"=w88, "Process"=w99, "ROI Descriptor"=w96, "Step Size"=w101, "Search Direction"=w97, "error in (no error)"=w95, "Edge Options"=w100) -> ("Edge Points-Array"=w102:cluster{"X":sgl, "Y":sgl}[][], "First Edges"=w86:T32[], "Last Edges"=w85:T32[], "Search Lines"=w78:T33[], "error out"=w87:errorcluster)  [unwired: 4 in]
          n7 = case shown="2, 3, Default" w97 {
            tunnel: [enum16{"Horizontal", "Vertical"}."Horizontal" ("Search Direction") enum16{"Horizontal", "Vertical"}."Vertical" ("Search Direction")] -> w103
            tunnel: [w105 w107] -> w98
            tunnel: w87 -> [w105 w107]
            frame 0, 1 {
            }
            frame 2, 3, Default {
            }
          }
          n8 = Array Size(array=w86) -> (size(s)=w93:i32)
          n9 = Divide(x=w93, y=2) -> (x/y=w92:dbl)
          n10 = Index Array(array=w78, index=w92) -> (element=w89:T33)
          n11 = Unbundle By Name(w89) -> ("Start Point"=w80:cluster{"X":sgl, "Y":sgl}, "End Point"=w79:cluster{"X":sgl, "Y":sgl})
          n12 = Index Array(array=w86, index=w92) -> (element=w91:T32)
          n13 = Index Array(array=w85, index=w92) -> (element=w90:T32)
          n14 = Unbundle By Name(w91) -> ("Location (Pixel)"=w84:cluster{"X":sgl, "Y":sgl})
          n15 = Unbundle By Name(w90) -> ("Location (Pixel)"=w83:cluster{"X":sgl, "Y":sgl})
          n16 = Build Array(w80, w79) -> ()  [unwired: 1 out]
          n17 = Bundle("Start Point"=w80, "Location (Pixel)"=w84, "Location (Pixel)"=w83, "End Point"=w79) -> (w82:T34)  [unwired: 1 in]
          n18 = Cluster To Array(cluster=w82) -> (array=w81:cluster{"X":sgl, "Y":sgl}[])
        }
        frame "Max" {
          n19 = Bundle By Name(cluster=T13 {"Contrast"=40, "Filter width"=4, "Steepness"=2, "Subsampling Ratio"=5, "Show Search Area"=FALSE, "Show Search Lines"=FALSE, "Show Edges Found"=FALSE, "Show Result"=FALSE} ("Settings"), "Subsampling Ratio"=w119) -> (w118:T13)
          n20 = call "IMAQ Convert ROI to Rectangle"("error in (no error)"=w114, "ROI Descriptor"=w117) -> ("error out"=w115:errorcluster, "Rectangle"=w116:T35)  [unwired: 7 in]
          n21 = case shown="0, 1, Default" w127 {
            tunnel: w126 -> [w155 w185]
            tunnel: [w154 w184] -> w125
            tunnel: w124 -> [w156 w183]
            tunnel: w116 -> [w150 w179]
            tunnel: [w153 w182] -> w123
            tunnel: [enum16{"Horizontal", "Vertical"}."Horizontal" ("Search Direction") enum16{"Horizontal", "Vertical"}."Vertical" ("Search Direction")] -> w121
            tunnel: w118 -> [w151 w180]
            tunnel: w115 -> [w149 w178]
            tunnel: [w130 w160] -> w113
            tunnel: [w137 w162] -> w112
            tunnel: [w136 w161] -> w111
            tunnel: [w128 w158] -> w110
            tunnel: [w128 w158] -> w109
            tunnel: [w129 w157] -> _
            frame 0, 1, Default {
              w145 = cluster{"X":sgl, "Y":sgl} {"X"=0.0, "Y"=0.0} ("element")
              n22 = call "Clamp AET Max_Horizontal.vi"("Image"=w155, "Rectangle"=w150, "error in (no error)"=w149, "Settings"=w151, "Edge Options"=w156) -> ("Edge Coordinates"=w129:cluster{"X":sgl, "Y":sgl}[], "Search Lines"=w128:T33[], "First Edges"=w137:T32[], "Last Edges"=w136:T32[], "error out"=w154:errorcluster)  [unwired: 7 in, 3 out]
              n23 = Index Array(array=w129, index #1=0 ("index"), index #2=1 ("index")) -> (element #1=w134:cluster{"X":sgl, "Y":sgl}, element #2=w133:cluster{"X":sgl, "Y":sgl})
              n24 = Unbundle By Name(w134) -> ("X"=w143:sgl, "Y"=w138:sgl)
              n25 = Unbundle By Name(w133) -> ("X"=w141:sgl, "Y"=w139:sgl)
              n26 = Subtract(x=w143, y=sgl 60.0) -> (x-y=w142:sgl)
              n27 = Add(x=w141, y=sgl 60.0) -> (x+y=w140:sgl)
              n28 = Bundle By Name(cluster=w145, "X"=w142, "Y"=w138) -> (w135:cluster{"X":sgl, "Y":sgl})
              n29 = Bundle By Name(cluster=w145, "X"=w140, "Y"=w139) -> (w132:cluster{"X":sgl, "Y":sgl})
              n30 = Bundle("element"=w135, w134, w133, "element"=w132) -> (w131:T36)  [unwired: 1 in]
              n31 = Cluster To Array(cluster=w131) -> (array=w130:cluster{"X":sgl, "Y":sgl}[])
              n32 = Build Array(w129) -> (w153:cluster{"X":sgl, "Y":sgl}[][])
            }
            frame 2, 3 {
              w172 = cluster{"X":sgl, "Y":sgl} {"X"=0.0, "Y"=0.0} ("element")
              n33 = call "Clamp AET Max_Vertical.vi"("Image"=w185, "Rectangle"=w179, "error in (no error)"=w178, "Settings"=w180, "Edge Options"=w183) -> ("Edge Coordinates"=w157:cluster{"X":sgl, "Y":sgl}[], "Search Lines"=w158:T33[], "First Edges"=w162:T32[], "Last Edges"=w161:T32[], "error out"=w184:errorcluster)  [unwired: 7 in, 3 out]
              n34 = Index Array(array=w157, index #1=0 ("index"), index #2=1 ("index")) -> (element #1=w173:cluster{"X":sgl, "Y":sgl}, element #2=w170:cluster{"X":sgl, "Y":sgl})
              n35 = Unbundle By Name(w173) -> ("X"=w166:sgl, "Y"=w168:sgl)
              n36 = Unbundle By Name(w170) -> ("X"=w163:sgl, "Y"=w165:sgl)
              n37 = Subtract(x=w168, y=sgl 60.0) -> (x-y=w167:sgl)
              n38 = Add(x=w165, y=sgl 60.0) -> (x+y=w164:sgl)
              n39 = Bundle By Name(cluster=w172, "X"=w166, "Y"=w167) -> (w174:cluster{"X":sgl, "Y":sgl})
              n40 = Bundle By Name(cluster=w172, "X"=w163, "Y"=w164) -> (w159:cluster{"X":sgl, "Y":sgl})
              n41 = Bundle("element"=w174, w173, w170, "element"=w159) -> (w169:T36)  [unwired: 1 in]
              n42 = Cluster To Array(cluster=w169) -> (array=w160:cluster{"X":sgl, "Y":sgl}[])
              n43 = Build Array(w157) -> (w182:cluster{"X":sgl, "Y":sgl}[][])
            }
          }
        }
        frame "Min" {
          n44 = Bundle By Name(cluster=T13 {"Contrast"=40, "Filter width"=4, "Steepness"=2, "Subsampling Ratio"=5, "Show Search Area"=FALSE, "Show Search Lines"=FALSE, "Show Edges Found"=FALSE, "Show Result"=TRUE} ("Settings"), "Subsampling Ratio"=w196) -> (w197:T13)
          n45 = call "IMAQ Convert ROI to Rectangle"("error in (no error)"=w193, "ROI Descriptor"=w191) -> ("error out"=w190:errorcluster, "Rectangle"=w195:T35)  [unwired: 7 in]
          n46 = case shown="0, 1" w204 {
            tunnel: [w227 w258] -> w202
            tunnel: w201 -> [w233 w256]
            tunnel: w200 -> [w232 w260]
            tunnel: [w231 w262] -> w199
            tunnel: w197 -> [w230 w261]
            tunnel: w195 -> [w228 w259]
            tunnel: w190 -> [w229 w257]
            tunnel: [enum16{"Horizontal", "Vertical"}."Vertical" ("Search Direction") enum16{"Horizontal", "Vertical"}."Horizontal" ("Search Direction")] -> w194
            tunnel: [w207 w236] -> w192
            tunnel: [w209 w238] -> w189
            tunnel: [w208 w237] -> w188
            tunnel: [w205 w234] -> w187
            tunnel: [w205 w234] -> w186
            frame 2, 3, Default {
              w220 = cluster{"X":sgl, "Y":sgl} {"X"=0.0, "Y"=0.0} ("element")
              n47 = call "Clamp AET Min_Vertical.vi"("Image"=w233, "Rectangle"=w228, "error in (no error)"=w229, "Settings"=w230, "Edge Options"=w232) -> ("First Edges 2"=w208:T32[], "Edge Coordinates"=w206:cluster{"X":sgl, "Y":sgl}[], "Search Lines"=w205:T33[], "First Edges"=w209:T32[], "error out"=w231:errorcluster)  [unwired: 6 in, 4 out]
              n48 = Index Array(array=w206, index #1=0 ("index"), index #2=1 ("index")) -> (element #1=w221:cluster{"X":sgl, "Y":sgl}, element #2=w218:cluster{"X":sgl, "Y":sgl})
              n49 = Unbundle By Name(w221) -> ("X"=w214:sgl, "Y"=w216:sgl)
              n50 = Unbundle By Name(w218) -> ("X"=w211:sgl, "Y"=w213:sgl)
              n51 = Subtract(x=w216, y=sgl 60.0) -> (x-y=w215:sgl)
              n52 = Add(x=w213, y=sgl 60.0) -> (x+y=w212:sgl)
              n53 = Bundle By Name(cluster=w220, "X"=w214, "Y"=w215) -> (w222:cluster{"X":sgl, "Y":sgl})
              n54 = Bundle By Name(cluster=w220, "X"=w211, "Y"=w212) -> (w217:cluster{"X":sgl, "Y":sgl})
              n55 = Bundle("element"=w222, w221, w218, "element"=w217) -> (w210:T36)  [unwired: 1 in]
              n56 = Cluster To Array(cluster=w210) -> (array=w207:cluster{"X":sgl, "Y":sgl}[])
              n57 = Build Array(w206) -> (w227:cluster{"X":sgl, "Y":sgl}[][])
            }
            frame 0, 1 {
              w249 = cluster{"X":sgl, "Y":sgl} {"X"=0.0, "Y"=0.0} ("element")
              n58 = call "Clamp AET Min_Horizontal.vi"("Image"=w256, "Rectangle"=w259, "error in (no error)"=w257, "Settings"=w261, "Edge Options"=w260) -> ("First Edges 2"=w237:T32[], "Edge Coordinates"=w235:cluster{"X":sgl, "Y":sgl}[], "Search Lines"=w234:T33[], "First Edges"=w238:T32[], "error out"=w262:errorcluster)  [unwired: 6 in, 4 out]
              n59 = Index Array(array=w235, index #1=0 ("index"), index #2=1 ("index")) -> (element #1=w250:cluster{"X":sgl, "Y":sgl}, element #2=w247:cluster{"X":sgl, "Y":sgl})
              n60 = Unbundle By Name(w250) -> ("X"=w245:sgl, "Y"=w240:sgl)
              n61 = Unbundle By Name(w247) -> ("X"=w243:sgl, "Y"=w241:sgl)
              n62 = Subtract(x=w245, y=sgl 60.0) -> (x-y=w244:sgl)
              n63 = Add(x=w243, y=sgl 60.0) -> (x+y=w242:sgl)
              n64 = Bundle By Name(cluster=w249, "X"=w244, "Y"=w240) -> (w251:cluster{"X":sgl, "Y":sgl})
              n65 = Bundle By Name(cluster=w249, "X"=w242, "Y"=w241) -> (w246:cluster{"X":sgl, "Y":sgl})
              n66 = Bundle("element"=w251, w250, w247, "element"=w246) -> (w239:T36)  [unwired: 1 in]
              n67 = Cluster To Array(cluster=w239) -> (array=w236:cluster{"X":sgl, "Y":sgl}[])
              n68 = Build Array(w235) -> (w258:cluster{"X":sgl, "Y":sgl}[][])
            }
          }
        }
      }
      n69 = Unbundle By Name(w13) -> ("OverlayROI"=w27:bool, "OverlayRakeLine"=w28:bool, "OverlayPoints"=w29:bool)
      n70 = case shown="True" w27 {
        tunnel: w15 -> [_ w51]
        tunnel: w26 -> [_ w50]
        frame False {
        }
        frame True {
          n71 = call "IMAQ Overlay ROI"("Colors (Green)"=u32[] [65280], "ROI Descriptor"=w51, "Image"=w50) -> ()  [unwired: 7 in, 2 out]
        }
      }
      n72 = call "Correction.vi"("Calibrated Image"=w37, "Vertical/Horizontal"=w43, "Algo Type"=w38, "appended array"=w44, "error in (no error)"=w48) -> ("Mesurement Value"=w39:sgl, "error IO"=w33:errorcluster)  [unwired: 8 in, 1 out]
      n73 = case shown="True" w28 {
        tunnel: w34 -> [_ w56]
        tunnel: w26 -> [_ w55]
        tunnel: w33 -> [w52 w54]
        tunnel: [w52 w53] -> w31
        frame False {
        }
        frame True {
          n74 = for {
            tunnel: w56 -> [w63] mode=indexing
            tunnel: w55 -> [w60]
            tunnel: w54 -> [w58]
            tunnel: [w57] -> w53
            n75 = Unbundle By Name(w63) -> ("Start Point"=w62:cluster{"X":sgl, "Y":sgl}, "End Point"=w61:cluster{"X":sgl, "Y":sgl})
            n76 = call "IMAQ Overlay Line"("Color"=u32 9567230, "error in (no error)"=w58, "End Point"=w61, "Start Point"=w62, "Image"=w60) -> ("error out"=w57:errorcluster)  [unwired: 5 in, 1 out]
          }
        }
      }
      n77 = case shown="True" w29 {
        tunnel: w36 -> [_ w74]
        tunnel: w35 -> [_ w73]
        tunnel: w26 -> [_ w69]
        tunnel: w33 -> [w64 w66]
        tunnel: [w64 w65] -> w32
        frame False {
        }
        frame True {
          n78 = Build Array (concatenate)(w74, w73) -> (w72:T32[])
          n79 = for {
            tunnel: w72 -> [w77] mode=indexing
            tunnel: [w76] -> w71 mode=indexing
            tunnel: [w75] -> w67
            tunnel: w66 -> [w75]
            n80 = Unbundle By Name(w77) -> ("Location (Pixel)"=w76:cluster{"X":sgl, "Y":sgl})
          }
          n81 = call "Overlay Points with User Specified Size.vi"("Color"=u32 16775281, "error in"=w67, "Point Diameter (5)"=u32 10, "Points"=w71, "Image In"=w69) -> ("error out"=w65:errorcluster)  [unwired: 5 in, 1 out]
        }
      }
      n82 = Index Array(array=w23) -> (element #1=w22:cluster{"X":sgl, "Y":sgl}, element #2=w21:cluster{"X":sgl, "Y":sgl}, element #3=w20:cluster{"X":sgl, "Y":sgl}, element #4=w19:cluster{"X":sgl, "Y":sgl})  [unwired: 4 in]
      n83 = Bundle("element"=w22, "element"=w21) -> (w18:T37)  [unwired: 1 in]
      n84 = Bundle("element"=w20, "element"=w19) -> (w17:T37)  [unwired: 1 in]
      n85 = Bundle By Name(cluster=T11 {"First Overlay Line "={"Start Point"={"X"=0.0, "Y"=0.0}, "Start Point"={"X"=0.0, "Y"=0.0}}, "Second Overlay Line "={"Start Point"={"X"=0.0, "Y"=0.0}, "Start Point"={"X"=0.0, "Y"=0.0}}}, "First Overlay Line"=w18, "Second Overlay Line"=w17) -> (w24:T11)
      n86 = Merge Errors(w31, w32) -> (w30:errorcluster)
    }
    frame "TT Width" {
      n87 = Unbundle By Name(w265) -> ("New Reference"=w264:T38)
      n88 = Unbundle By Name(w275) -> ("Ref ROI Cluster.ROI Ref"=w274:T39, "Measurement ROI 1 Cluster.Meas ROI 1"=w273:T2, "Ref ROI Cluster.Edge Options ROI Ref"=w272:T5, "Ref ROI Cluster.Line Options ROI Ref"=w271:T7, "Ref ROI Cluster.Search Direction ROI Ref"=w270:u32, "Measurement ROI 1 Cluster.Step Size ROI 1"=w269:u32, "Measurement ROI 1 Cluster.Edge Options ROI 1"=w268:T5, "Measurement ROI 1 Cluster.Scan/Search Direction ROI 1"=w267:u16, "Measurement ROI 1 Cluster.Process ROI 1"=w266:T24)
      n89 = Unbundle By Name(w264) -> ("Origin"=w263:cluster{"X":sgl, "Y":sgl})
      n90 = Bundle By Name(cluster=T14 {"AvgMinMax"=enum."Average", "Center X &Y"={"Center X"=0.0, "Center Y"=0.0}, "Reference ROI Before Transformation"={"Global Rectangle"=[], "Contours"=[]}, "Measurement ROI-1 Before transformation"={"Global Rectangle"=[], "Contours"=[]}, "Ref Line Edge Options"={"Edge Polarity"=0, "Kernel Size"=0, "Width"=0, "Minimum Edge Strength"=0.0, "Interpolation Type"=enum."Zero Order", "Data Processing Method"=enum."Average"}, "Ref Line Search Direction"=0, "Ref Line Options"={"Number of Lines"=0, "Type"=enum."First Edge Rake", "Min. Score"=0.0, "Max. Score"=0.0, "Orientation"=0.0, "Angle Range"=0.0, "Angle Tolerance"=0.0, "Step Size"=0, "Min. SNR (db)"=0.0, "Min. Points (%)"=0.0, "Hough Iterations"=0}, "Meas ROI-1 Edge Options"={"Edge Polarity"=0, "Kernel Size"=0, "Width"=0, "Minimum Edge Strength"=0.0, "Interpolation Type"=enum."Zero Order", "Data Processing Method"=enum."Average"}, "Meas ROI-1 Step Size"=0, "Meas ROI-1 Scan Direction"=0, "Meas ROI-1 Process"=enum."Get First Edge", "OverlayOptions"={"OverlayEnable"=FALSE, "OverlayText"="", "OverlayCoords"=[], "OverlayAngle"=0, "OverlayTextSize"=0, "OverlayTextColor"="", "OverlayROI"=FALSE, "OverlayRakeLine"=FALSE, "OverlayPoints"=FALSE}} ("TT side Width Input Cluster"), "AvgMinMax"=enum16{"Average", "Max", "Min", "Max2"}."Max", "Center X &Y"=w263, "Reference ROI Before Transformation"=w274, "Measurement ROI-1 Before transformation"=w273, "Ref Line Edge Options"=w272, "Ref Line Search Direction"=w270, "Ref Line Options"=w271, "Meas ROI-1 Edge Options"=w268, "Meas ROI-1 Step Size"=w269, "Meas ROI-1 Scan Direction"=w267, "Meas ROI-1 Process"=w266) -> (w277:T14)
      n91 = call "TT_Width.vi"("Calibrated Image in"=w283, "error in (no error)"=w279, "TT side Width Input Cluster"=w277, "Image In"=w284) -> ("error out"=w282:errorcluster, "Measurement 1"=w281:sgl, "Overlay Arrow Lines"=w280:T11)  [unwired: 3 in, 2 out]
    }
    frame "Linear Length 1" {
      n92 = Unbundle By Name(w309) -> ("Measurement ROI 1 Cluster.Edge Options ROI 1"=w300:T5, "Measurement ROI 1 Cluster.Scan/Search Direction ROI 1"=w299:u16, "Measurement ROI 1 Cluster.Line Options ROI 1"=w301:T7, "Measurement ROI 2 Cluster.Step Size ROI 2"=w298:u32, "Measurement ROI 2 Cluster.Process ROI 2"=w297:T24, "Measurement ROI 2 Cluster.Edge Options ROI 2"=w296:T5, "Measurement ROI 2 Cluster.Scan/Search Direction ROI 2"=w295:u32, "OverlayOptions"=w292:T31)
      n93 = Unbundle By Name(w287) -> ("Measurement ROI 1 [After Transformation]"=w286:T2, "Measurement ROI 2 [After Transformation]"=w285:T2)
      n94 = Unbundle By Name(w292) -> ("OverlayROI"=w290:bool, "OverlayRakeLine"=w289:bool, "OverlayPoints"=w291:bool)
      n95 = Bundle By Name(cluster=T16 {"ROI 1 Descriptor"={"Global Rectangle"=[], "Contours"=[]}, "ROI 1 Line Options"={"Number of Lines"=1, "Type"=enum."Best Edge Rake", "Min. Score"=10.0, "Max. Score"=1000.0, "Orientation"=0.0, "Angle Range"=10.0, "Angle Tolerance"=1.0, "Step Size"=5, "Min. SNR (db)"=0.0, "Min. Points (%)"=25.0, "Hough Iterations"=5}, "ROI 1 Edge Options"={"Edge Polarity"=2, "Kernel Size"=3, "Width"=3, "Minimum Edge Strength"=25.0, "Interpolation Type"=enum."Zero Order", "Data Processing Method"=enum."Average"}, "ROI 1 Search Direction"=1, "ROI 1 Overlay"=TRUE, "ROI 1 Rake Line Overlay"=TRUE, "ROI 1 Edge/Point Overlay"=TRUE} ("ROI 1 Parameters"), "ROI 1 Descriptor"=w286, "ROI 1 Line Options"=w301, "ROI 1 Edge Options"=w300, "ROI 1 Search Direction"=w299, "ROI 1 Overlay"=w290, "ROI 1 Rake Line Overlay"=w289, "ROI 1 Edge/Point Overlay"=w291) -> (w294:T16)
      n96 = Bundle By Name(cluster=T15 {"ROI 2 Descriptor"={"Global Rectangle"=[], "Contours"=[]}, " ROI 2 Step Size"=10, "ROI 2 Scan Direction"=0, "ROI 2 Process"=enum."Get First + Last Edge", "ROI 2 Edge Options"={"Edge Polarity"=0, "Kernel Size"=3, "Width"=3, "Minimum Edge Strength"=40.0, "Interpolation Type"=enum."Zero Order", "Data Processing Method"=enum."Average"}, "ROI 2 Overlay"=TRUE, "ROI 2 Rake Line Overlay"=TRUE, "ROI 2 Edge/Point Overlay"=TRUE} ("ROI 2 Parameters"), "ROI 2 Descriptor"=w285, "ROI 2 Step Size"=w298, "ROI 2 Scan Direction"=w295, "ROI 2 Process"=w297, "ROI 2 Edge Options"=w296, "ROI 2 Overlay"=w290, "ROI 2 Rake Line Overlay"=w289, "ROI 2 Edge/Point Overlay"=w291) -> (w293:T15)
      n97 = call "Linear Length 1 1721 1853.vi"("Calibration Image"=w305, "error in"=w306, "ROI 2 Parameters"=w293, "ROI 1 Parameters"=w294, "Input Image"=w304) -> ("error  out"=w308:errorcluster, "Overlay Arrow Lines"=w288:T11, "L Outputs"=w307:T40)  [unwired: 2 in, 1 out]
      n98 = Unbundle By Name(w307) -> ("L"=w310:dbl)
    }
    frame "Linear Length 2" {
      n99 = Unbundle By Name(w343) -> ("Ref ROI Cluster.Edge Options ROI Ref"=w334:T5, "Ref ROI Cluster.Line Options ROI Ref"=w333:T7, "Ref ROI Cluster.Search Direction ROI Ref"=w332:u32, "Measurement ROI 1 Cluster.Edge Options ROI 1"=w331:T5, "Measurement ROI 1 Cluster.Scan/Search Direction ROI 1"=w330:u16, "Measurement ROI 1 Cluster.Step Size ROI 1"=w329:u32, "Measurement ROI 1 Cluster.Process ROI 1"=w328:T24, "Measurement ROI 2 Cluster.Edge Options ROI 2"=w327:T5, "Measurement ROI 2 Cluster.Scan/Search Direction ROI 2"=w326:u32, "Measurement ROI 2 Cluster.Step Size ROI 2"=w325:u32, "Measurement ROI 2 Cluster.Process ROI 2"=w324:T24, "OverlayOptions"=w319:T31)
      n100 = Unbundle By Name(w314) -> ("ROI Ref [ After Transformation]"=w313:T2, "Measurement ROI 1 [After Transformation]"=w312:T2, "Measurement ROI 2 [After Transformation]"=w311:T2)
      n101 = Bundle By Name(cluster=T19 {"Ref ROI After Transformation"={"Global Rectangle"=[], "Contours"=[]}, "Ref ROI Edge Options"={"Edge Polarity"=0, "Kernel Size"=3, "Width"=3, "Minimum Edge Strength"=10.0, "Interpolation Type"=enum."Zero Order", "Data Processing Method"=enum."Average"}, "Ref ROI Line Options"={"Number of Lines"=1, "Type"=enum."Best Edge Projection", "Min. Score"=0.0, "Max. Score"=1000.0, "Orientation"=0.0, "Angle Range"=5.0, "Angle Tolerance"=0.0, "Step Size"=5, "Min. SNR (db)"=0.0, "Min. Points (%)"=25.0, "Hough Iterations"=5}, "Ref ROI Search Direction"=0, "Ref ROI Overlay"=FALSE} ("Ref ROI Parameters"), "Ref ROI After Transformation"=w313, "Ref ROI Edge Options"=w334, "Ref ROI Line Options"=w333, "Ref ROI Search Direction"=w332, "Ref ROI Overlay"=TRUE) -> (w323:T19)
      n102 = Unbundle By Name(w319) -> ("OverlayROI"=w317:bool, "OverlayRakeLine"=w318:bool, "OverlayPoints"=w316:bool)
      n103 = Bundle By Name(cluster=T18 {"ROI 1 After Transformation"={"Global Rectangle"=[], "Contours"=[]}, "ROI 1 Edge Options"={"Edge Polarity"=0, "Kernel Size"=3, "Width"=3, "Minimum Edge Strength"=10.0, "Interpolation Type"=enum."Bilinear Fixed", "Data Processing Method"=enum."Average"}, "ROI 1 Scan Direction"=0, "ROI 1 Step Size"=0, "ROI 1 Process"=enum."Get First Edge", "ROI 1 Overlay"=FALSE, "ROI 1 Rake Line Overlay"=FALSE, "ROI 1 Edge/Point Overlay"=FALSE} ("ROI 1 Parameters"), "ROI 1 After Transformation"=w312, "ROI 1 Edge Options"=w331, "ROI 1 Scan Direction"=w330, "ROI 1 Step Size"=w329, "ROI 1 Process"=w328, "ROI 1 Overlay"=w317, "ROI 1 Rake Line Overlay"=w316, "ROI 1 Edge/Point Overlay"=w316) -> (w322:T18)
      n104 = Bundle By Name(cluster=T17 {"ROI 2 After Transformation"={"Global Rectangle"=[], "Contours"=[]}, "ROI 2 Edge Options"={"Edge Polarity"=0, "Kernel Size"=3, "Width"=3, "Minimum Edge Strength"=10.0, "Interpolation Type"=enum."Bilinear Fixed", "Data Processing Method"=enum."Average"}, "ROI 2 Scan Direction"=0, "ROI 2 Step Size"=0, "ROI 2 Process"=enum."Get First Edge", "ROI 2 Overlay"=FALSE, "ROI 2 Rake Line Overlay"=FALSE, "ROI 2 Edge/Point Overlay"=FALSE} ("ROI 2 Parameters"), "ROI 2 After Transformation"=w311, "ROI 2 Edge Options"=w327, "ROI 2 Scan Direction"=w326, "ROI 2 Step Size"=w325, "ROI 2 Process"=w324, "ROI 2 Overlay"=w317, "ROI 2 Rake Line Overlay"=w318, "ROI 2 Edge/Point Overlay"=w316) -> (w321:T17)
      n105 = call "Linear Length 2 1478 1525 1828.vi"("Input Image"=w342, "Calibration Image"=w341, "Ref ROI Parameters"=w323, "ROI 1 Parameters"=w322, "ROI 2 Parameters"=w321, "error in (no error)"=w340) -> ("output cluster"=w338:T41, "Overlay Arrow Lines"=w315:T42, "error out"=w339:errorcluster)  [unwired: 6 in, 1 out]
      n106 = Unbundle By Name(w338) -> ("L Meas"=w344:sgl)
    }
    frame "Lancing Presence 2" {
      n107 = Unbundle By Name(w381) -> ("Measurement ROI 1 Cluster.Edge Options ROI 1"=w379:T5, "Measurement ROI 1 Cluster.Line Options ROI 1"=w378:T7, "Measurement ROI 1 Cluster.Scan/Search Direction ROI 1"=w377:u16, "Measurement ROI 2 Cluster.Edge Options ROI 2"=w376:T5, "Measurement ROI 2 Cluster.Scan/Search Direction ROI 2"=w374:u32, "Measurement ROI 2 Cluster.Step Size ROI 2"=w375:u32, "Measurement ROI 2 Cluster.Process ROI 2"=w373:T24)
      n108 = Unbundle By Name(w347) -> ("Measurement ROI 1 [After Transformation]"=w346:T2, "Measurement ROI 2 [After Transformation]"=w345:T2)
      n109 = Bundle By Name(cluster=T23 {"Search Direction"=3, "Edge Options"={"Edge Polarity"=2, "Kernel Size"=5, "Width"=5, "Minimum Edge Strength"=50.0, "Interpolation Type"=enum."Zero Order", "Data Processing Method"=enum."Average"}, "Show Search Area"=FALSE, "Show Search Lines"=FALSE, "Show Edges Found"=TRUE, "Show Result"=TRUE, "Search Area Color"=65280, "Search Lines Color"=255, "Edge Locations Color"=16776960, "Result Color"=16711680, "Overlay Group Name"=""} ("Options"), "Search Direction"=w377, "Edge Options"=w379, "Show Search Area"=TRUE, "Show Search Lines"=TRUE, "Show Edges Found"=TRUE, "Show Result"=FALSE) -> (w383:T23)
      n110 = call "IMAQ Overlay ROI"("Colors (Green)"=u32[] [13816530], "ROI Descriptor"=w345, "Image"=w353) -> ()  [unwired: 7 in, 2 out]
      n111 = call "IMAQ Find Edge"("Line Fit Options"=w378, "Options"=w383, "error in (no error)"=w380, "ROI Descriptor"=w346, "Image"=w353) -> ("error out"=w410:errorcluster, "Straight Edges"=w412:T43)  [unwired: 3 in, 2 out]
      n112 = call "IMAQ Rake 3"("Image"=w353, "Edge Options"=w376, "ROI Descriptor"=w345, "Step Size"=w375, "Scan Direction"=w374, "error in (no error)"=w410, "Process"=w373) -> ("First Edges"=w408:T32[], "error out"=w402:errorcluster)  [unwired: 5 in, 2 out]
      n113 = for {
        tunnel: w408 -> [w414] mode=indexing
        tunnel: [w413] -> w409 mode=indexing
        n114 = Unbundle By Name(w414) -> ("Distance (Pixel)"=w413:dbl)
      }
      n115 = Array Max & Min(array=w409) -> (min index (indices)=w407:i32)  [unwired: 3 out]
      n116 = Index Array(array=w412) -> (element=w411:T44)  [unwired: 1 in]
      n117 = Unbundle By Name(w411) -> ("Point1 (Pixels)"=w405:cluster{"X":sgl, "Y":sgl}, "Point2 (Pixels)"=w404:cluster{"X":sgl, "Y":sgl})
      n118 = Index Array(array=w408, index=w407) -> (element=w406:T32)
      n119 = Unbundle By Name(w406) -> ("Location (Pixel)"=w401:cluster{"X":sgl, "Y":sgl})
      n120 = Bundle("Point1 (Pixels)"=w405, "Point2 (Pixels)"=w404) -> (w403:T45)  [unwired: 1 in]
      n121 = call "IMAQ Perpendicular Line"("error in (no error)"=w402, "Point"=w401, "Line"=w403) -> ("error out"=w382:errorcluster, "Perpendicular Line"=w399:T46)  [unwired: 6 in, 1 out]
      n122 = call "IMAQ Overlay Points"("Color"=u32 16711680, "Point"=w401, "Image"=w353) -> ()  [unwired: 7 in, 2 out]
      n123 = Unbundle By Name(w399) -> ("Point 1"=w349:cluster{"X":sgl, "Y":sgl}, "Point 2"=w348:cluster{"X":sgl, "Y":sgl})
      n124 = Unbundle By Name(w349) -> ("X"=w359:sgl, "Y"=w358:sgl)
      n125 = Build Array(w349, w348) -> (w397:cluster{"X":sgl, "Y":sgl}[])
      n126 = Build Array(w349, w348) -> (w394:cluster{"X":sgl, "Y":sgl}[])
      n127 = Unbundle By Name(w348) -> ("X"=w367:sgl, "Y"=w366:sgl)
      n128 = call "IMAQ Overlay Line"("Color"=u32 1244159, "End Point"=w348, "Start Point"=w349, "Image"=w353) -> ()  [unwired: 6 in, 2 out]
      n129 = call "IMAQ Point Distances"("Points"=w397) -> ("Distances"=w396:sgl[])  [unwired: 4 in, 1 out]
      n130 = call "IMAQ Convert Pixel to Real World"("error in (no error)"=w382, "Array of Pixel Coordinates"=w394, "Calibrated Image"=w354) -> ("error out"=w355:errorcluster, "Array of Real World Coordinates"=w393:cluster{"X":sgl, "Y":sgl}[])  [unwired: 3 in, 4 out]
      n131 = Subtract(x=w358, y=sgl 30.0) -> (x-y=w362:sgl)
      n132 = Add(x=w366, y=sgl 30.0) -> (x+y=w364:sgl)
      n133 = Index Array(array=w396) -> (element=→"Pixel Value":sgl)  [unwired: 1 in]
      n134 = Index Array(array=w393) -> (element #1=w391:cluster{"X":sgl, "Y":sgl}, element #2=w390:cluster{"X":sgl, "Y":sgl})  [unwired: 2 in]
      n135 = Bundle By Name(cluster=cluster{"X":sgl, "Y":sgl} {"X"=0.0, "Y"=0.0} ("Start Point"), "X"=w359, "Y"=w362) -> (w357:cluster{"X":sgl, "Y":sgl})
      n136 = Bundle By Name(cluster=cluster{"X":sgl, "Y":sgl} {"X"=0.0, "Y"=0.0} ("Start Point"), "X"=w367, "Y"=w364) -> (w363:cluster{"X":sgl, "Y":sgl})
      n137 = Build Array(w391, w390) -> (w389:cluster{"X":sgl, "Y":sgl}[])
      n138 = call "IMAQ Point Distances"("Points"=w389) -> ("Distances"=w392:sgl[])  [unwired: 4 in, 1 out]
      n139 = Bundle By Name(cluster=T21 {"Start Point"={"X"=0.0, "Y"=0.0}, "Point 1"={"X"=0.0, "Y"=0.0}} ("First Overlay Line"), "Start Point"=w357, "Point 1"=w348) -> (w351:T21)
      n140 = Bundle By Name(cluster=T20 {"Point 2"={"X"=0.0, "Y"=0.0}, "Start Point"={"X"=0.0, "Y"=0.0}} ("Second Overlay Line"), "Point 2"=w349, "Start Point"=w363) -> (w350:T20)
      n141 = Index Array(array=w392) -> (element=w372:sgl)  [unwired: 1 in]
      "Real World Value" <- w372
      n142 = Bundle By Name(cluster=T22 {"First Overlay Line "={"Start Point"={"X"=0.0, "Y"=0.0}, "Point 1"={"X"=0.0, "Y"=0.0}}, "Second Overlay Line "={"Point 2"={"X"=0.0, "Y"=0.0}, "Start Point"={"X"=0.0, "Y"=0.0}}} ("Arrow Overlay lines"), "First Overlay Line"=w351, "Second Overlay Line"=w350) -> (w356:T22)
    }
    frame "Circlular_Dia", Default {
      w443 = cluster{"X":sgl, "Y":sgl} {"X"=0.0, "Y"=0.0} ("Center (Pixels)")
      n143 = Unbundle By Name(w416) -> ("Measurement ROI 1 [After Transformation]"=w415:T2)
      n144 = Unbundle By Name(w432) -> ("Measurement ROI 1 Cluster.Circle Options ROI 1"=w420:T47, "Measurement ROI 1 Cluster.Circle Fit Options ROI 1"=w431:T10, "OverlayOptions.OverlayROI"=w422:bool, "OverlayOptions.OverlayRakeLine"=w418:bool, "OverlayOptions.OverlayPoints"=w417:bool)
      "Circle Fit Options ROI 1" <- w431
      n145 = call "ConvertRectangularROI2AnnularROI.vi"("error in (no error)"=w436, "ROI"=w415) -> ("error out"=w452:errorcluster, "Annulus"=w451:T48)  [unwired: 8 in]
      n146 = Bundle By Name(cluster=w420, "Show Search Lines"=w418, "Show Edges Found"=w417) -> (w419:T47)
      n147 = call "IMAQ Convert Annulus to ROI"("error in (no error)"=w452, "Annulus"=w451) -> ("error out"=w450:errorcluster, "ROI Descriptor"=w424:T2)  [unwired: 7 in]
      n148 = case shown="True" w422 {
        tunnel: w424 -> [_ w457]
        tunnel: w421 -> [_ w456]
        tunnel: w421 -> [_ w454]
        tunnel: w415 -> [_ w453]
        frame False {
        }
        frame True {
          n149 = call "IMAQ Overlay ROI"("Colors (Green)"=u32[] [3381759], "ROI Descriptor"=w457, "Image"=w456) -> ()  [unwired: 7 in, 2 out]
          n150 = call "IMAQ Overlay ROI"("Colors (Green)"=u32[] [3381759], "ROI Descriptor"=w453, "Image"=w454) -> ()  [unwired: 7 in, 2 out]
        }
      }
      n151 = call "IMAQ Find Circular Edge 3"("Circle Fit Options"=w431, "Options"=w419, "error in (no error)"=w450, "ROI Descriptor"=w424, "Image"=w421) -> ("error out"=w439:errorcluster, "Fitted Circle"=w449:T49)  [unwired: 2 in, 3 out]
      n152 = Unbundle By Name(w449) -> ("Center (Pixels)"=w448:cluster{"X":sgl, "Y":sgl}, "Radius (Pixels)"=w445:dbl)
      n153 = Unbundle By Name(w448) -> ("X"=w446:sgl, "Y"=w442:sgl)
      n154 = Add(x=w446, y=w445) -> (x+y=w447:dbl)
      n155 = Subtract(x=w446, y=w445) -> (x-y=w444:dbl)
      n156 = Bundle By Name(cluster=w443, "X"=w447, "Y"=w442) -> (w428:cluster{"X":sgl, "Y":sgl})
      n157 = Bundle By Name(cluster=w443, "X"=w444, "Y"=w442) -> (w429:cluster{"X":sgl, "Y":sgl})
      n158 = Bundle("Center (Pixels)"=w429, "Center (Pixels)"=w428) -> (w427:T50)  [unwired: 1 in]
      n159 = Bundle("Center (Pixels)"=w429, "Center (Pixels)"=w428) -> (w426:T50)  [unwired: 1 in]
      n160 = Bundle("Center (Pixels)"=w428, "Center (Pixels)"=w429) -> (w434:T50)  [unwired: 1 in]
      n161 = Bundle(w427, w426) -> (w425:T51)  [unwired: 1 in]
      n162 = Cluster To Array(cluster=w434) -> (array=w430:cluster{"X":sgl, "Y":sgl}[])
      n163 = call "IMAQ Convert Pixel to Real World"("error in (no error)"=w439, "Array of Pixel Coordinates"=w430, "Calibrated Image"=w423) -> ("error out"=w438:errorcluster, "Array of Real World Coordinates"=w441:cluster{"X":sgl, "Y":sgl}[])  [unwired: 3 in, 4 out]
      n164 = call "IMAQ Point Distances"("Points"=w441, "error in (no error)"=w438) -> ("Distances"=w440:sgl[], "error out"=w433:errorcluster)  [unwired: 3 in]
      n165 = Index Array(array=w440, index=0) -> (element=w435:sgl)
    }
    frame "Front" {
      n166 = Unbundle By Name(w481) -> ("Ref ROI Cluster.ROI Ref"=w468:T39, "Ref ROI Cluster.Edge Options ROI Ref"=w478:T5, "Ref ROI Cluster.Search Direction ROI Ref"=w473:u32, "Measurement ROI 1 Cluster.Edge Options ROI 1"=w477:T5, "Measurement ROI 1 Cluster.Step Size ROI 1"=w476:u32, "Measurement ROI 1 Cluster.Process ROI 1"=w475:T24, "Measurement ROI 1 Cluster.Scan/Search Direction ROI 1"=w474:u16, "Measurement ROI 1 Cluster.Meas ROI 1"=w461:T2, "OverlayOptions.OverlayEnable"=w460:bool)
      n167 = Unbundle By Name(w469) -> ("Front Reference center 2"=w465:cluster{"X":sgl, "Y":sgl}, "Front Angle"=w459:dbl)
      n168 = Unbundle By Name(w465) -> ("X"=w464:sgl, "Y"=w463:sgl)
      n169 = call "IMAQ Convert ROI to Rectangle"("ROI Descriptor"=w468) -> ("Rectangle"=w467:T35)  [unwired: 8 in, 1 out]
      n170 = call "IMAQ Convert ROI to Rectangle"("ROI Descriptor"=w461) -> ("Rectangle"=w462:T35)  [unwired: 8 in, 1 out]
      n171 = call "Dhoot Front Measurement Block.vi"("Image in"=w480, "Coord Centre X"=w464, "Measurement ROI"=w462, "Coord Centre Y"=w463, "Angle"=w459, "ROI Enable"=w460, "error in (no error)"=w466, "Measurement ROI Scan Direction"=w474, "Measurement Reference ROI"=w467, "Measu ROI Process"=w475, "Measu ROI Step Size"=w476, "Measu Ref Edge Options"=w478, "Measu Edge Options"=w477, "Measu Ref Scan Direction"=w473, "Calibration Image"=w479) -> ("Overlay Arrows Lines"=w470:T11, "Measurement"=w471:sgl, "error IO"=w472:errorcluster)  [unwired: 5 in, 5 out]
    }
    frame "Curl Height" {
      n172 = Unbundle By Name(w507) -> ("Ref ROI Cluster.Search Direction ROI Ref"=w504:u32, "Ref ROI Cluster.Edge Options ROI Ref"=w503:T5, "Ref ROI Cluster.ROI Ref"=w489:T39, "OverlayOptions.OverlayEnable"=w502:bool, "Measurement ROI 1 Cluster.Meas ROI 1"=w488:T2, "Measurement ROI 1 Cluster.Edge Options ROI 1"=w501:T5, "Measurement ROI 1 Cluster.Step Size ROI 1"=w500:u32, "Measurement ROI 1 Cluster.Process ROI 1"=w499:T24, "Measurement ROI 1 Cluster.Scan/Search Direction ROI 1"=w498:u16)
      n173 = Unbundle By Name(w486) -> ("Front Angle"=w485:dbl, "Front Reference center 2"=w484:cluster{"X":sgl, "Y":sgl})
      n174 = Unbundle By Name(w484) -> ("X"=w483:sgl, "Y"=w482:sgl)
      n175 = call "IMAQ Convert ROI to Rectangle"("ROI Descriptor"=w489) -> ("Rectangle"=w490:T35)  [unwired: 8 in, 1 out]
      n176 = call "IMAQ Convert ROI to Rectangle"("ROI Descriptor"=w488) -> ("Rectangle"=w487:T35)  [unwired: 8 in, 1 out]
      n177 = Build Array(w484) -> (w494:cluster{"X":sgl, "Y":sgl}[])
      n178 = call "Curl Height.vi"("Image in"=w492, "Coord Centre X"=w483, "Coord Centre Y"=w482, "Angle"=w485, "Overlay Enable"=w502, "Measurement ROI"=w487, "Measu Edge Options"=w501, "error in (no error)"=w506, "Measurement Reference ROI"=w490, "Measu ROI Step Size"=w500, "Measu Ref Edge Options"=w503, "Measu ROI Process"=w499, "Measu Ref Scan Direction"=w504, "Measurement ROI Scan Direction"=w498, "Calibrated Image in"=w505) -> ("Overlay Arrows Line"=w495:T11, "Curl Height"=w497:dbl, "error out"=w496:errorcluster)  [unwired: 7 in, 3 out]
      n179 = call "Overlay Points with User Specified Size.vi"("Color"=u32 16711680, "Point Diameter (5)"=u32 20, "Points"=w494, "Image In"=w492) -> ()  [unwired: 6 in, 2 out]
    }
    frame "Side Horizontal" {
      n180 = Unbundle By Name(w531) -> ("Measurement ROI 1 Cluster.Meas ROI 1"=w528:T2, "Ref ROI Cluster.Edge Options ROI Ref"=w527:T5, "Measurement ROI 1 Cluster.Edge Options ROI 1"=w526:T5, "Ref ROI Cluster.Search Direction ROI Ref"=w525:u32, "Measurement ROI 1 Cluster.Scan/Search Direction ROI 1"=w524:u16, "Ref ROI Cluster.Line Options ROI Ref"=w522:T7, "Measurement ROI 1 Cluster.Step Size ROI 1"=w521:u32, "Measurement ROI 1 Cluster.Process ROI 1"=w520:T24, "OverlayOptions"=w519:T31)
      n181 = Unbundle By Name(w509) -> ("ROI Ref [ After Transformation]"=w508:T2)
      n182 = Unbundle By Name(w519) -> ("OverlayROI"=w517:bool, "OverlayRakeLine"=w518:bool, "OverlayPoints"=w516:bool)
      n183 = call "Side Horizontal.vi"("Image In"=w530, "Ref ROI Descriptor"=w508, "ROI 1"=w528, "Edge Options Ref ROI"=w527, "Edge Options ROI 1"=w526, "Ref ROI Search Direction"=w525, "Search Direction ROI 1"=w524, "error in (no error)"=w523, "Calib Image"=w529, "Line Options Ref ROI"=w522, "Step Size ROI 1"=w521, "Process ROI 1"=w520, "Overlay ROI"=w517, "Overlay Rake Lines"=w518, "Overlay Points"=w516) -> ("First Overlay Line"=w514:T52, "Second Overlay Line"=w513:T53, "Mesurement Value"=w512:sgl, "error out"=w511:errorcluster)  [unwired: 9 in]
      n184 = Bundle By Name(cluster=T22 {"First Overlay Line "={"Start Point"={"X"=0.0, "Y"=0.0}, "Point 1"={"X"=0.0, "Y"=0.0}}, "Second Overlay Line "={"Point 2"={"X"=0.0, "Y"=0.0}, "Start Point"={"X"=0.0, "Y"=0.0}}} ("Arrow Overlay lines"), "First Overlay Line"=w514, "Second Overlay Line"=w513) -> (w510:T22)
    }
    frame "Point to Point" {
      n185 = Unbundle By Name(w537) -> ("Algo Type"=w536:string)
      n186 = call "Point to Point VI.vi"("Measurement Type"=w536, "CalibratedImage In"=w538, "error in (no error)"=w540, "Transformed ROI cluster"=w535, "Measurement JSON Data"=w537, "Image In"=w539) -> ("error out"=w533:errorcluster, "Measurement Value"=w532:sgl, "Overlay Arrow Lines"=w534:T22)  [unwired: 3 in]
    }
    frame "Twist Angle" {
      w557 = u16 2 items=["Left To Right", "Right To Left", "Top To Bottom", "Bottom To Top"] ("Scan Direction")
      # "code modified (20-07-2018)\noverlay disabled"
      n187 = Unbundle By Name(w541) -> ("Measurement ROI 1 [After Transformation]"=w560:T2)
      n188 = Subtract(x=sgl 0.0, y=sgl 0.903062) -> (x-y=w547:sgl)
      n189 = case shown="False" TRUE {
        tunnel: w561 -> [w591 _]
        tunnel: w560 -> [w590 _]
        frame False {
          n190 = call "IMAQ Overlay ROI"("Colors (Green)"=u32[] [16773418], "ROI Descriptor"=w590, "Image"=w591) -> ()  [unwired: 7 in, 2 out]
        }
        frame True {
        }
      }
      n191 = Absolute Value(x=w547) -> (abs(x)=w546:sgl)
      n192 = Divide(x=w546, y=sgl 0.03) -> ()  [unwired: 1 out]
      n193 = call "IMAQ Rake 3"("Image"=w561, "Edge Options"=T5 {"Edge Polarity"=0, "Kernel Size"=7, "Width"=7, "Minimum Edge Strength"=50.0, "Interpolation Type"=enum."Bilinear Fixed", "Data Processing Method"=enum."Average"}, "ROI Descriptor"=w560, "Step Size"=u32 2, "Scan Direction"=w557, "error in (no error)"=w549, "Process"=T24."Get First + Last Edge") -> ("First Edges"=w556:T32[], "Last Edges"=w555:T32[], "error out"=w550:errorcluster)  [unwired: 5 in, 1 out]
      n194 = for {
        tunnel: w556 -> [w601] mode=indexing
        tunnel: w555 -> [w600] mode=indexing
        tunnel: [w594] -> w563 mode=indexing if=w593
        n195 = Unbundle By Name(w601) -> ("Location (Pixel)"=w599:cluster{"X":sgl, "Y":sgl})
        n196 = Unbundle By Name(w600) -> ("Location (Pixel)"=w598:cluster{"X":sgl, "Y":sgl})
        n197 = Build Array(w599, w598) -> (w597:cluster{"X":sgl, "Y":sgl}[])
        n198 = call "IMAQ Point Distances"("Points"=w597) -> ("Distances"=w596:sgl[])  [unwired: 4 in, 1 out]
        n199 = Index Array(array=w596) -> (element=w594:sgl)  [unwired: 1 in]
        n200 = Not Equal?(x=w594, y=0.0) -> (x != y?=w593:bool)
      }
      n201 = Array Max & Min(array=w563) -> (min index (indices)=w543:i32)  [unwired: 3 out]
      n202 = Index Array(array=w556, index=w543) -> (element=w554:T32)
      n203 = Index Array(array=w555, index=w543) -> (element=w553:T32)
      n204 = Unbundle By Name(w554) -> ("Location (Pixel)"=w552:cluster{"X":sgl, "Y":sgl})
      n205 = Unbundle By Name(w553) -> ("Location (Pixel)"=w551:cluster{"X":sgl, "Y":sgl})
      n206 = Unbundle By Name(w552) -> ("X"=w579:sgl, "Y"=w578:sgl)
      n207 = Unbundle By Name(w551) -> ("X"=w575:sgl, "Y"=w574:sgl)
      n208 = call "IMAQ Convert Pixel to Real World"("error in (no error)"=w550, "Pixel Coordinates"=w552, "Calibrated Image"=w589) -> ("error out"=w583:errorcluster, "Real World Coordinates"=w588:cluster{"X":sgl, "Y":sgl})  [unwired: 3 in, 4 out]
      n209 = call "IMAQ Convert Pixel to Real World"("error in (no error)"=w550, "Pixel Coordinates"=w551, "Calibrated Image"=w589) -> ("error out"=w582:errorcluster, "Real World Coordinates"=w587:cluster{"X":sgl, "Y":sgl})  [unwired: 3 in, 4 out]
      n210 = Merge Errors(w583, w582) -> (w581:errorcluster)
      n211 = Build Array(w588, w587) -> (w586:cluster{"X":sgl, "Y":sgl}[])
      n212 = Subtract(x=w578, y=sgl 30.0) -> (x-y=w576:sgl)
      n213 = Add(x=w574, y=sgl 30.0) -> (x+y=w572:sgl)
      n214 = call "IMAQ Point Distances"("Points"=w586, "error in (no error)"=w581) -> ("Distances"=w585:sgl[], "error out"=w580:errorcluster)  [unwired: 3 in]
      n215 = Bundle("X"=w579, w576) -> (w568:cluster{"X":sgl, sgl})  [unwired: 1 in]
      n216 = Bundle("X"=w575, w572) -> (w567:cluster{"X":sgl, sgl})  [unwired: 1 in]
      n217 = Index Array(array=w585) -> (element=w545:sgl)  [unwired: 1 in]
      n218 = Bundle By Name(cluster=T21 {"Start Point"={"X"=0.0, "Y"=0.0}, "Point 1"={"X"=0.0, "Y"=0.0}} ("First Overlay Line"), "Start Point"=w568, "Point 1"=w552) -> (w566:T21)
      n219 = Bundle By Name(cluster=T20 {"Point 2"={"X"=0.0, "Y"=0.0}, "Start Point"={"X"=0.0, "Y"=0.0}} ("Second Overlay Line"), "Point 2"=w551, "Start Point"=w567) -> (w565:T20)
      n220 = Bundle By Name(cluster=T22 {"First Overlay Line "={"Start Point"={"X"=0.0, "Y"=0.0}, "Point 1"={"X"=0.0, "Y"=0.0}}, "Second Overlay Line "={"Point 2"={"X"=0.0, "Y"=0.0}, "Start Point"={"X"=0.0, "Y"=0.0}}} ("Arrow Overlay lines"), "First Overlay Line"=w566, "Second Overlay Line"=w565) -> (w564:T22)
    }
    frame "Lancing 2" {
      n221 = Unbundle By Name(w620) -> ("ROI Ref [ After Transformation]"=w615:T2, "Measurement ROI 1 [After Transformation]"=w624:T2)
      n222 = Unbundle By Name(w619) -> ("Measurement ROI 1 Cluster"=w617:T54, "Measurement ROI 2 Cluster"=w616:T55, "OverlayOptions"=w609:T31, "Ref ROI Cluster"=w605:T56)
      n223 = Unbundle By Name(w616) -> ("Edge Options ROI 2"=w606:T5, "Scan/Search Direction ROI 2"=w610:u32, "Step Size ROI 2"=w607:u32, "Process ROI 2"=w608:T24)
      n224 = Unbundle By Name(w616) -> ("Meas ROI 2"=w618:T2)
      n225 = Unbundle By Name(w605) -> ("Edge Options ROI Ref"=w604:T5, "Line Options ROI Ref"=w602:T7, "Search Direction ROI Ref"=w603:u32)
      n226 = Unbundle By Name(w617) -> ("Edge Options ROI 1"=w612:T5, "Scan/Search Direction ROI 1"=w613:u16, "Step Size ROI 1"=w614:u32, "Process ROI 1"=w611:T24)
      n227 = call "Lancing 2 Integ.vi"("Image Out"=w625, "REF ROI"=w615, "Edge Options Ref ROI"=w604, "Search Direction Ref ROI"=w603, "Line Options Ref ROI"=w602, "Meas ROI 1"=w624, "Meas ROI 2"=w618, "error in (no error)"=w623, "Calibrated Image"=w626, "Edge Options ROI 1"=w612, "Step Size ROI 1"=w614, "Process ROI 1"=w611, "Scan Direction ROI 1"=w613, "Process ROI 2"=w608, "Step Size ROI 2"=w607, "OverlayOptions"=w609, "Edge Options ROI 2"=w606, "Scan Direction ROI 2"=w610) -> ("Lancing 2"=w621:sgl, "error out"=w622:errorcluster)  [unwired: 8 in]
    }
    frame "Front Gap" {
      n228 = Unbundle By Name(w632) -> ("Measurement ROI 1 [After Transformation]"=w631:T2, "Measurement ROI 2 [After Transformation]"=w630:T2)
      n229 = call "Motherson Gap algorithm int.vi"("Image Out"=w635, "Calibrated Image"=w634, "ROI 1"=w631, "ROI 2"=w630, "error in (no error)"=w633) -> ("Gap"=w627:sgl, "output cluster"=w628:T57, "error out"=w629:errorcluster)  [unwired: 12 in]
    }
    frame "Linear Length 3" {
      n230 = Unbundle By Name(w657) -> ("ROI Ref [ After Transformation]"=w654:T2, "Measurement ROI 1 [After Transformation]"=w653:T2, "Measurement ROI 2 [After Transformation]"=w650:T2)
      n231 = Unbundle By Name(w649) -> ("Ref ROI Cluster"=w641:T56, "Measurement ROI 1 Cluster"=w648:T54, "Measurement ROI 2 Cluster"=w647:T55)
      n232 = Unbundle By Name(w641) -> ("Edge Options ROI Ref"=w640:T5, "Line Options ROI Ref"=w638:T7, "Search Direction ROI Ref"=w639:u32)
      n233 = Unbundle By Name(w647) -> ("Edge Options ROI 2"=w636:T5, "Scan/Search Direction ROI 2"=w645:u32, "Step Size ROI 2"=w644:u32, "Process ROI 2"=w643:T24)
      n234 = Unbundle By Name(w648) -> ("Edge Options ROI 1"=w637:T5, "Line Options ROI 1"=w646:T7, "Scan/Search Direction ROI 1"=w642:u16)
      n235 = call "terminal_length_integrated.vi"("ROI Ref"=w654, "Edge Options ROI Ref"=w640, "Search Direction ROI Ref"=w639, "Line Options ROI Ref"=w638, "ROI 1"=w653, "Edge Options ROI 1"=w637, "Search Direction ROI 1"=w642, "error in (no error)"=w659, "Image In"=w656, "Line Options ROI 1"=w646, "Calibrated Image"=w655, "Edge Options ROI 2"=w636, "ROI 2"=w650, "Scan Direction ROI 2"=w645, "Process ROI 2"=w643, "Step Size ROI 2"=w644) -> ("overlay arrow lines"=w651:T58, "Terminal Length"=w652:sgl, "error out"=w658:errorcluster)  [unwired: 9 in]
    }
    frame "Terminal Angle" {
      n236 = Unbundle By Name(w666) -> ("Measurement ROI 1 Cluster.Edge Options ROI 1"=w665:T5, "Measurement ROI 1 Cluster.Line Options ROI 1"=w664:T7, "Measurement ROI 1 Cluster.Scan/Search Direction ROI 1"=w663:u16, "OverlayOptions"=w662:T31)
      n237 = Unbundle By Name(w668) -> ("ROI Ref [ After Transformation]"=w667:T2)
      n238 = call "Terminal Angle Side view int.vi"("Image"=w670, "Search Direction ROI 1"=w663, "ROI Descriptor"=w667, "Edge Options ROI 1"=w665, "Line Options ROI 1"=w664, "error in (no error)"=w669, "OverlayOptions"=w662) -> ("Angle"=w660:sgl, "error out"=w661:errorcluster)  [unwired: 7 in]
    }
    frame "XY Position" {
      n239 = Unbundle By Name(w681) -> ("Measurement ROI 1 [After Transformation]"=w680:T2)
      n240 = Unbundle By Name(w679) -> ("Measurement ROI 1 Cluster"=w678:T54, "OverlayOptions"=w671:T31)
      n241 = Unbundle By Name(w678) -> ("Edge Options ROI 1"=w677:T5, "Line Options ROI 1"=w676:T7, "Scan/Search Direction ROI 1"=w675:u16)
      n242 = call "x_pos_y_pos_int.vi"("Image Out"=w682, "Calibrated Image"=w683, "ROI Descriptor"=w680, "Edge Options ROI 1"=w677, "Search Direction ROI 1"=w675, "error in (no error)"=w674, "Line Options ROI 1"=w676, "OverlayOptions"=w671) -> ("Position"=w673:sgl, "error out"=w672:errorcluster)  [unwired: 6 in]
    }
    frame "Y Position" {
      n243 = Unbundle By Name(w699) -> ("Base Reference"=w698:T38, "New Reference"=w693:T38)
      n244 = Unbundle By Name(w698) -> ("Origin"=w697:cluster{"X":sgl, "Y":sgl})
      n245 = Unbundle By Name(w693) -> ("Origin"=w694:cluster{"X":sgl, "Y":sgl})
      n246 = call "IMAQ Convert Pixel to Real World"("error in (no error)"=w689, "Pixel Coordinates"=w697, "Calibrated Image"=w685) -> ("error out"=w688:errorcluster, "Real World Coordinates"=w696:cluster{"X":sgl, "Y":sgl})  [unwired: 3 in, 4 out]
      n247 = call "IMAQ Convert Pixel to Real World"("error in (no error)"=w688, "Pixel Coordinates"=w694, "Calibrated Image"=w685) -> ("error out"=w686:errorcluster, "Real World Coordinates"=w695:cluster{"X":sgl, "Y":sgl})  [unwired: 3 in, 4 out]
      n248 = Unbundle By Name(w696) -> ("Y"=w692:sgl)
      n249 = Unbundle By Name(w695) -> ("Y"=w691:sgl)
      n250 = Subtract(x=w692, y=w691) -> (x-y=w690:sgl)
      n251 = Absolute Value(x=w690) -> (abs(x)=w687:sgl)
    }
    frame "X Position" {
      n252 = Unbundle By Name(w715) -> ("Base Reference"=w714:T38, "New Reference"=w709:T38)
      n253 = Unbundle By Name(w714) -> ("Origin"=w713:cluster{"X":sgl, "Y":sgl})
      n254 = Unbundle By Name(w709) -> ("Origin"=w710:cluster{"X":sgl, "Y":sgl})
      n255 = call "IMAQ Convert Pixel to Real World"("error in (no error)"=w705, "Pixel Coordinates"=w713, "Calibrated Image"=w701) -> ("error out"=w704:errorcluster, "Real World Coordinates"=w712:cluster{"X":sgl, "Y":sgl})  [unwired: 3 in, 4 out]
      n256 = call "IMAQ Convert Pixel to Real World"("error in (no error)"=w704, "Pixel Coordinates"=w710, "Calibrated Image"=w701) -> ("error out"=w702:errorcluster, "Real World Coordinates"=w711:cluster{"X":sgl, "Y":sgl})  [unwired: 3 in, 4 out]
      n257 = Unbundle By Name(w712) -> ("X"=w708:sgl)
      n258 = Unbundle By Name(w711) -> ("X"=w707:sgl)
      n259 = Subtract(x=w708, y=w707) -> (x-y=w706:sgl)
      n260 = Absolute Value(x=w706) -> (abs(x)=w703:sgl)
    }
    frame "Side E" {
      n261 = Unbundle By Name(w754) -> ("New Reference"=w753:T38)
      n262 = Unbundle By Name(w744) -> ("Ref ROI Cluster"=w743:T56, "Measurement ROI 1 Cluster"=w735:T54, "OverlayOptions"=w738:T31)
      n263 = Unbundle By Name(w738) -> ("OverlayROI"=w734:bool, "OverlayRakeLine"=w733:bool, "OverlayPoints"=w732:bool)
      n264 = Unbundle By Name(w753) -> ("Origin"=w752:cluster{"X":sgl, "Y":sgl})
      n265 = Unbundle By Name(w743) -> ("ROI Ref"=w742:T39, "Edge Options ROI Ref"=w740:T5, "Line Options ROI Ref"=w739:T7, "Search Direction ROI Ref"=w741:u32)
      n266 = case shown="\"Min\"" w746 {
        tunnel: [enum16{"Average", "Max", "Min", "Max2"}."Max" ("AvgMinMax 2") enum16{"Average", "Max", "Min", "Max2"}."Min" ("AvgMinMax 2") enum16{"Average", "Max", "Min", "Max2"}."Average" ("AvgMinMax 2")] -> w745
        frame "Max", Default {
        }
        frame "Min" {
        }
        frame "Average" {
        }
      }
      n267 = Bundle By Name(cluster=T28 {"Ref Line ROI Before Transformation"={"Global Rectangle"=[], "Contours"=[]}, "Ref ROI Search Direction"=2, "Ref ROI Edge Options"={"Edge Polarity"=2, "Kernel Size"=3, "Width"=3, "Minimum Edge Strength"=50.0, "Interpolation Type"=enum."Zero Order", "Data Processing Method"=enum."Average"}, "Ref ROI Line Options"={"Number of Lines"=1, "Type"=enum."Best Edge Rake", "Min. Score"=10.0, "Max. Score"=1000.0, "Orientation"=0.0, "Angle Range"=10.0, "Angle Tolerance"=10.0, "Step Size"=14, "Min. SNR (db)"=0.0, "Min. Points (%)"=25.0, "Hough Iterations"=5}, "Ref ROI Overlay"=FALSE, "Ref Rake Line Overlay 2"=FALSE, "Ref Edge/Point Overlay"=FALSE} ("Ref ROI Parameters"), "Ref Line ROI Before Transformation"=w742, "Ref ROI Search Direction"=w741, "Ref ROI Edge Options"=w740, "Ref ROI Line Options"=w739, "Ref ROI Overlay"=w734, "Ref Rake Line Overlay 2"=w733, "Ref Edge/Point Overlay"=w732) -> (w747:T28)
      n268 = Unbundle By Name(w735) -> ("Meas ROI 1"=w731:T2, "Edge Options ROI 1"=w730:T5, "Scan/Search Direction ROI 1"=w729:u16, "Step Size ROI 1"=w728:u32, "Process ROI 1"=w727:T24)
      n269 = Bundle By Name(cluster=T27 {"ROI 1 Before Transformation"={"Global Rectangle"=[], "Contours"=[]}, "ROI 1 Scan Direction"=0, "ROI 1 Edge Options"={"Edge Polarity"=0, "Kernel Size"=3, "Width"=3, "Minimum Edge Strength"=50.0, "Interpolation Type"=enum."Zero Order", "Data Processing Method"=enum."Average"}, "ROI 1Step Size"=3, "ROI 1 Process"=enum."Get First + Last Edge", "ROI 1 Overlay"=FALSE, "ROI 1 Rake Line Overlay"=FALSE, "ROI 1 Edge/Point Overlay"=FALSE} ("Measurement ROI Parameters"), "ROI 1 Before Transformation"=w731, "ROI 1 Scan Direction"=w729, "ROI 1 Edge Options"=w730, "ROI 1Step Size"=w728, "ROI 1 Process"=w727, "ROI 1 Overlay"=w734, "ROI 1 Rake Line Overlay"=w733, "ROI 1 Edge/Point Overlay"=w732) -> (w736:T27)
      n270 = call "Side E.vi"("Input Image"=w749, "Calibrated Image"=w750, "Ref ROI Parameters"=w747, "Measurement ROI Parameters"=w736, "AvgMinMax 2"=w745, "error in (no error)"=w751, "Center X &Y"=w752) -> ("output cluster"=w726:T59, "error out"=w725:errorcluster)  [unwired: 6 in, 1 out]
      n271 = Unbundle By Name(w726) -> ("E Side EMeasurement"=w724:sgl, "Points for Arrow Overlay"=w723:cluster{"X":sgl, "Y":sgl}[])
      n272 = Index Array(array=w723) -> (element #1=w722:cluster{"X":sgl, "Y":sgl}, element #2=w721:cluster{"X":sgl, "Y":sgl}, element #3=w720:cluster{"X":sgl, "Y":sgl}, element #4=w719:cluster{"X":sgl, "Y":sgl})  [unwired: 4 in]
      n273 = Bundle("End Point"=w722, "End Point"=w721) -> (w718:T60)  [unwired: 1 in]
      n274 = Bundle("End Point"=w720, "End Point"=w719) -> (w717:T60)  [unwired: 1 in]
      n275 = Bundle(w718, w717) -> (w716:T61)  [unwired: 1 in]
    }
    frame "Side Vertical Minimum" {
      w780 = cluster{"X":sgl, "Y":sgl} {"X"=0.0, "Y"=0.0} ("element")
      n276 = Unbundle By Name(w791) -> ("Ref ROI Cluster"=w803:T56)
      n277 = Unbundle By Name(w791) -> ("OverlayOptions.OverlayROI"=w790:bool, "OverlayOptions.OverlayRakeLine"=w789:bool, "OverlayOptions.OverlayPoints"=w788:bool)
      n278 = Unbundle By Name(w791) -> ("Measurement ROI 1 Cluster"=w802:T54)
      n279 = Unbundle By Name(w803) -> ("ROI Ref"=w801:T39, "Edge Options ROI Ref"=w797:T5, "Line Options ROI Ref"=w796:T7, "Search Direction ROI Ref"=w798:u32)
      n280 = Unbundle By Name(w805) -> ("New Reference.Origin"=w804:cluster{"X":sgl, "Y":sgl})
      n281 = Unbundle By Name(w802) -> ("Meas ROI 1"=w787:T2, "Edge Options ROI 1"=w795:T5, "Step Size ROI 1"=w793:u32)  [unwired: 2 out]
      n282 = Bundle By Name(cluster=T29 {"Overlay ROI"=TRUE, "Overlay Edge/ Points"=TRUE, "Overlay Rake Lines"=TRUE} ("Overlay Boolean Cluster"), "Overlay ROI"=w790, "Overlay Edge/ Points"=w788, "Overlay Rake Lines"=w789) -> (w786:T29)
      n283 = call "Ref_ROI_Translated_From_Ellipse_Center.vi"("Ellipse Center"=w804, "ROI Descriptor"=w801) -> ("Traslated ROI"=w800:T62)  [unwired: 9 in]
      n284 = Unbundle By Name(w795) -> ("Minimum Edge Strength"=w794:sgl)
      n285 = call "IMAQ Convert Rectangle to ROI"("Rectangle"=w800) -> ("ROI Descriptor"=w799:T2)  [unwired: 8 in, 1 out]
      n286 = call "Side VErtical Minimum.vi"("Image"=w807, "Calibrated Image"=w806, "Ellipse Center"=w804, "Search Direction ROI Ref"=w798, "Edge Options ROI Ref"=w797, "error in (no error)"=w808, "ROI 1 Edge Strength"=w794, "Line Options ROI Ref"=w796, "Edge Options ROI 1"=w795, "Ref ROI after Transformation SV"=w799, "Meas ROI 1 Before Transformation"=w787, "ROI 1Step Size"=w793, "Overlay Boolean Cluster"=w786) -> ("Edge Coordinates"=w759:cluster{"X":sgl, "Y":sgl}[], "Numeric"=w785:sgl, "error out"=w784:errorcluster)  [unwired: 12 in]
      n287 = Index Array(array=w759, index #1=0 ("index"), index #2=1 ("index")) -> (element #1=w770:cluster{"X":sgl, "Y":sgl}, element #2=w778:cluster{"X":sgl, "Y":sgl})
      n288 = Unbundle By Name(w770) -> ("X"=w773:sgl, "Y"=w777:sgl)
      n289 = Unbundle By Name(w778) -> ("Y"=w760:sgl)
      n290 = Subtract(x=w777, y=sgl 60.0) -> (x-y=w776:sgl)
      n291 = Add(x=w760, y=sgl 60.0) -> (x+y=w775:sgl)
      n292 = Bundle By Name(cluster=cluster{"X":sgl, "Y":sgl} {"X"=0.0, "Y"=0.0} ("element"), "X"=w773, "Y"=w760) -> (w769:cluster{"X":sgl, "Y":sgl})
      n293 = Bundle By Name(cluster=w780, "X"=w773, "Y"=w776) -> (w771:cluster{"X":sgl, "Y":sgl})
      n294 = Bundle By Name(cluster=w780, "X"=w773, "Y"=w775) -> (w768:cluster{"X":sgl, "Y":sgl})
      n295 = Replace Array Subset(array=cluster{"X":sgl, "Y":sgl}[] [{"X"=0.0, "Y"=0.0}, {"X"=0.0, "Y"=0.0}, {"X"=0.0, "Y"=0.0}, {"X"=0.0, "Y"=0.0}] ("appended array"), new element #1=w771, new element #2=w770, new element #3=w769, new element #4=w768) -> (w767:cluster{"X":sgl, "Y":sgl}[])  [unwired: 4 in]
      n296 = Index Array(array=w767) -> (element #1=w766:cluster{"X":sgl, "Y":sgl}, element #2=w765:cluster{"X":sgl, "Y":sgl}, element #3=w764:cluster{"X":sgl, "Y":sgl}, element #4=w763:cluster{"X":sgl, "Y":sgl})  [unwired: 4 in]
      n297 = Bundle("element"=w766, "element"=w765) -> (w762:T37)  [unwired: 1 in]
      n298 = Bundle("element"=w764, "element"=w763) -> (w761:T37)  [unwired: 1 in]
      n299 = Bundle(w762, w761) -> (w758:T63)  [unwired: 1 in]
    }
    frame "Side Vertical Lancing" {
      n300 = Unbundle By Name(w829) -> ("Measurement ROI 1 Cluster.Meas ROI 1"=w816:T2, "Measurement ROI 1 Cluster.Edge Options ROI 1"=w813:T5, "Measurement ROI 1 Cluster.Scan/Search Direction ROI 1"=w817:u16, "Measurement ROI 1 Cluster.Step Size ROI 1"=w814:u32, "Measurement ROI 1 Cluster.Process ROI 1"=w815:T24)
      n301 = Unbundle By Name(w828) -> ("New Reference"=w827:T38)
      n302 = Unbundle By Name(w827) -> ("Origin"=w812:cluster{"X":sgl, "Y":sgl})
      n303 = Unbundle By Name(w829) -> ("Ref ROI Cluster.ROI Ref"=w826:T39, "Ref ROI Cluster.Edge Options ROI Ref"=w811:T5, "Ref ROI Cluster.Line Options ROI Ref"=w810:T7, "Ref ROI Cluster.Search Direction ROI Ref"=w809:u32)
      n304 = call "Ref_ROI_Translated_From_Ellipse_Center.vi"("Ellipse Center"=w812, "ROI Descriptor"=w826) -> ("Traslated ROI"=w825:T62)  [unwired: 9 in]
      n305 = call "IMAQ Convert Rectangle to ROI"("Rectangle"=w825) -> ("ROI Descriptor"=w824:T2)  [unwired: 8 in, 1 out]
      n306 = call "Side_Vertical_Lancing_Integrated.vi"("Image Out"=w822, "Ref ROI Search Direction"=w809, "Ref ROI Edge Options"=w811, "Ref ROI Line Options"=w810, "ROI 1 Edge Options"=w813, "ROI 1 Step Size"=w814, "ROI 1 Process"=w815, "error in (no error)"=w818, "Calibrated Image"=w823, "ROI 1 Scan Direction"=w817, "Ref ROI After SV Transformation"=w824, "Measurement ROI 1 Before Tranformation"=w816, "Ellipse Center"=w812) -> ("Overlay Arrow Lines"=w821:T64, "Measurement Lancing"=w819:sgl, "error out"=w820:errorcluster)  [unwired: 12 in]
    }
    frame "Side E1" {
      n307 = Unbundle By Name(w852) -> ("Ref ROI Cluster.ROI Ref"=w840:T39, "Ref ROI Cluster.Search Direction ROI Ref"=w841:u32, "Ref ROI Cluster.Edge Options ROI Ref"=w842:T5, "Ref ROI Cluster.Line Options ROI Ref"=w843:T7, "Measurement ROI 1 Cluster.Meas ROI 1"=w844:T2, "Measurement ROI 1 Cluster.Step Size ROI 1"=w845:u32, "Measurement ROI 1 Cluster.Scan/Search Direction ROI 1"=w846:u16, "Measurement ROI 1 Cluster.Edge Options ROI 1"=w847:T5, "Measurement ROI 2 Cluster.Meas ROI 2"=w848:T2, "Measurement ROI 2 Cluster.Scan/Search Direction ROI 2"=w849:u32, "Measurement ROI 2 Cluster.Edge Options ROI 2"=w850:T5, "Measurement ROI 2 Cluster.Line Options ROI 2"=w851:T7)
      n308 = Unbundle By Name(w858) -> ("New Reference.Origin"=w857:cluster{"X":sgl, "Y":sgl})
      n309 = Bundle By Name(cluster=T30 {"1629 side E Ref ROI before transformation"={"Global Rectangle"=[], "Contours"=[]}, "Ref Search Direction"=2, "Ref Edge Options"={"Edge Polarity"=2, "Kernel Size"=3, "Width"=3, "Minimum Edge Strength"=50.0, "Interpolation Type"=enum."Zero Order", "Data Processing Method"=enum."Average"}, "Ref Line Options"={"Number of Lines"=1, "Type"=enum."Best Edge Rake", "Min. Score"=10.0, "Max. Score"=1000.0, "Orientation"=0.0, "Angle Range"=10.0, "Angle Tolerance"=1.0, "Step Size"=3, "Min. SNR (db)"=0.0, "Min. Points (%)"=25.0, "Hough Iterations"=5}, "Meas ROI-1 Descriptor before transformation"={"Global Rectangle"=[], "Contours"=[]}, "Meas-1 Step Size"=5, "Meas-1 Scan Direction"=2, "Meas-1 Edge Options"={"Edge Polarity"=0, "Kernel Size"=3, "Width"=3, "Minimum Edge Strength"=50.0, "Interpolation Type"=enum."Zero Order", "Data Processing Method"=enum."Average"}, "Meas ROI-2 Descriptor Before Transformation"={"Global Rectangle"=[], "Contours"=[]}, "Meas-2 Scan Direction"=0, "Meas-2 Edge Options"={"Edge Polarity"=2, "Kernel Size"=3, "Width"=3, "Minimum Edge Strength"=50.0, "Interpolation Type"=enum."Zero Order", "Data Processing Method"=enum."Average"}, "Meas-2 Line Options"={"Number of Lines"=1, "Type"=enum."Best Edge Rake", "Min. Score"=10.0, "Max. Score"=1000.0, "Orientation"=0.0, "Angle Range"=10.0, "Angle Tolerance"=1.0, "Step Size"=3, "Min. SNR (db)"=0.0, "Min. Points (%)"=25.0, "Hough Iterations"=5}, "Ellipse Center"={"X"=0.0, "Y"=0.0}} ("1629_E1 inputs"), "1629 side E Ref ROI before transformation"=w840, "Ref Search Direction"=w841, "Ref Edge Options"=w842, "Ref Line Options"=w843, "Meas ROI-1 Descriptor before transformation"=w844, "Meas-1 Step Size"=w845, "Meas-1 Scan Direction"=w846, "Meas-1 Edge Options"=w847, "Meas ROI-2 Descriptor Before Transformation"=w848, "Meas-2 Scan Direction"=w849, "Meas-2 Edge Options"=w850, "Meas-2 Line Options"=w851, "Ellipse Center"=w857) -> (w853:T30)
      n310 = call "1629_Side E1.vi"("error in (no error)"=w854, "1629_E1 inputs"=w853, "Calibrated Image"=w856, "Input Image"=w855) -> ("error out"=w838:errorcluster, "1629_E1 outtput"=w860:T65)  [unwired: 5 in, 1 out]
      n311 = Unbundle By Name(w860) -> ("Points for Overlay"=w837:cluster{"X":sgl, "Y":sgl}[], "E1"=w839:sgl)
      n312 = Index Array(array=w837) -> (element #1=w836:cluster{"X":sgl, "Y":sgl}, element #2=w835:cluster{"X":sgl, "Y":sgl}, element #3=w834:cluster{"X":sgl, "Y":sgl}, element #4=w833:cluster{"X":sgl, "Y":sgl})  [unwired: 4 in]
      n313 = Bundle("Point 1"=w836, "Point 1"=w835) -> (w832:T66)  [unwired: 1 in]
      n314 = Bundle("Point 1"=w834, "Point 1"=w833) -> (w831:T66)  [unwired: 1 in]
      n315 = Bundle(w832, w831) -> (w830:T67)  [unwired: 1 in]
    }
    frame "Side Linear Length" {
      n316 = Unbundle By Name(w886) -> ("New Reference"=w868:T38)
      n317 = Unbundle By Name(w868) -> ("Origin.X"=w885:sgl, "Origin.Y"=w884:sgl)
      n318 = Unbundle By Name(w881) -> ("Measurement ROI 1 Cluster"=w882:T54)
      n319 = Unbundle By Name(w881) -> ("Measurement ROI 2 Cluster.Meas ROI 2"=w873:T2, "Measurement ROI 2 Cluster.Edge Options ROI 2"=w875:T5, "Measurement ROI 2 Cluster.Line Options ROI 2"=w874:T7, "Measurement ROI 2 Cluster.Scan/Search Direction ROI 2"=w872:u32, "Measurement ROI 2 Cluster.Step Size ROI 2"=w870:u32, "Measurement ROI 2 Cluster.Process ROI 2"=w871:T24)
      n320 = Unbundle By Name(w868) -> ("Origin"=w867:cluster{"X":sgl, "Y":sgl})
      n321 = Unbundle By Name(w881) -> ("Ref ROI Cluster"=w883:T56)
      n322 = Unbundle By Name(w882) -> ("Meas ROI 1"=w880:T2, "Edge Options ROI 1"=w876:T5, "Scan/Search Direction ROI 1"=w878:u16, "Step Size ROI 1"=w879:u32, "Process ROI 1"=w877:T24)  [unwired: 1 out]
      n323 = Unbundle By Name(w883) -> ("ROI Ref"=w866:T39, "Edge Options ROI Ref"=w864:T5, "Search Direction ROI Ref"=w869:u32)  [unwired: 1 out]
      n324 = call "Ref_ROI_Translated_From_Ellipse_Center.vi"("Ellipse Center"=w867, "ROI Descriptor"=w866) -> ("Traslated ROI"=w865:T62)  [unwired: 9 in]
      n325 = call "Dhoot_Sealed_side.vi"("Calibrated Image"=w887, "Image In"=w888, "Centre X"=w885, "Centre Y"=w884, "Ref Edge ROI"=w865, "Ref Search Direction"=w869, "Ref Edge Options"=w864, "error in (no error)"=w889, "Meas ROI 1 [Before Transformation]"=w880, "Ref Line Options"=w874, "ROI 1 Step Size"=w879, "Meas ROI 2 [Before Transformation]"=w873, "ROI 1 Scan Direction"=w878, "ROI 2 Step Size"=w870, "ROI 1 Process"=w877, "ROI 2 Scan Direction"=w872, "ROI 1 Edge Options"=w876, "ROI 2 Process"=w871, "ROI 2 Edge Options"=w875) -> ("Side Length"=w861:sgl, "Arrow Overlay lines"=w862:T68, "error out"=w863:errorcluster)  [unwired: 6 in]
    }
  }
  "error out" <- w8
  "Numeric" <- w9
  "Overlay Arrow Lines" <- w7
